vi "Check_Execution_Row.vi"(0 "Execution Row":T1 {"Carrier_2 Q (l/min)" format="%#.2f"; "Row Duration (mins)" format="%#.1f"; "Row No" min=0; "Trace Gas Concentration (%)" min=0.0 format="%#_4f"; "Carrier_1 Q (l/min)" format="%#.4f"; "Start X" format="%#.2f"; "Start Y" format="%#.2f"; "Start Z" format="%#.2f"; "End X" format="%#.2f"; "End Y" format="%#.2f"; "End Z" format="%#.2f"; "Tunnel Speed" format="%#.2f"; "Averaging time (mins)" min=0.0 format="%#.2f"}, 1 "Earlier Filenames":path[](array[path]), 2 "multirunFilepath":path, 3 "Synchronization Start No":i32=1 min=1 max=100, 4 "Row Index":i32, 5 "Max Tunnel Speed":dbl format="%.2f") -> (6 "Edited Row":bool, 7 "Execution Row Out":T1 {"Carrier_2 Q (l/min)" format="%#.2f"; "Row Duration (mins)" format="%#.1f"; "Row No" min=0; "Trace Gas Concentration (%)" min=0.0 format="%#_4f"; "Carrier_1 Q (l/min)" format="%#.4f"; "Start X" format="%#.2f"; "Start Y" format="%#.2f"; "Start Z" format="%#.2f"; "End X" format="%#.2f"; "End Y" format="%#.2f"; "End Z" format="%#.2f"; "Tunnel Speed" format="%#.2f"; "Averaging time (mins)" min=0.0 format="%#.2f"}, 9 "Continue?":bool, 10 "Error Comments":string)   [LabVIEW 2022 SP3]
uses:
  Traverse_cluster.ctl
  Spacing.ctl
  Controls/Multi_run_mode.ctl
  Controls/User_Specific_mode.ctl
  Controls/Home.ctl
  Controls/Tunnel_Coordinates.ctl
  ADAM Client/Sub VIs/ADAM Controls/Channel_names.ctl
  <vilib>/Utility/error.llb/Trim Whitespace One-Sided.vi
  Globals/Extra_Commands_Global.vi
  Globals/Constants_global.vi
  Globals/Trav_pos_global.vi
  Globals/Preference_global.vi
panel:
  out "Traverse line Out":T1 {"Carrier_2 Q (l/min)" format="%#.2f"; "Row Duration (mins)" format="%#.1f"; "Row No" min=0; "Trace Gas Concentration (%)" min=0.0 format="%#_4f"; "Carrier_1 Q (l/min)" format="%#.4f"; "Start X" format="%#.2f"; "Start Y" format="%#.2f"; "Start Z" format="%#.2f"; "End X" format="%#.2f"; "End Y" format="%#.2f"; "End Z" format="%#.2f"; "Tunnel Speed" format="%#.2f"; "Averaging time (mins)" min=0.0 format="%#.2f"}
  out "Fixed Axis":bool[](array[boolean])
  out "Filenames":string[](array[string])
  out "Current Sync Number":i32
  out "Checks":string[](array[string])
  in  "Edit in Excel":bool
  in  "OK":bool
  # "X           Y          Z"
  # "Start"
  # "End"
  # "X           Y          Z"
  # "Start"
  # "End"
  # "X           Y          Z"
  # "Start"
  # "End"
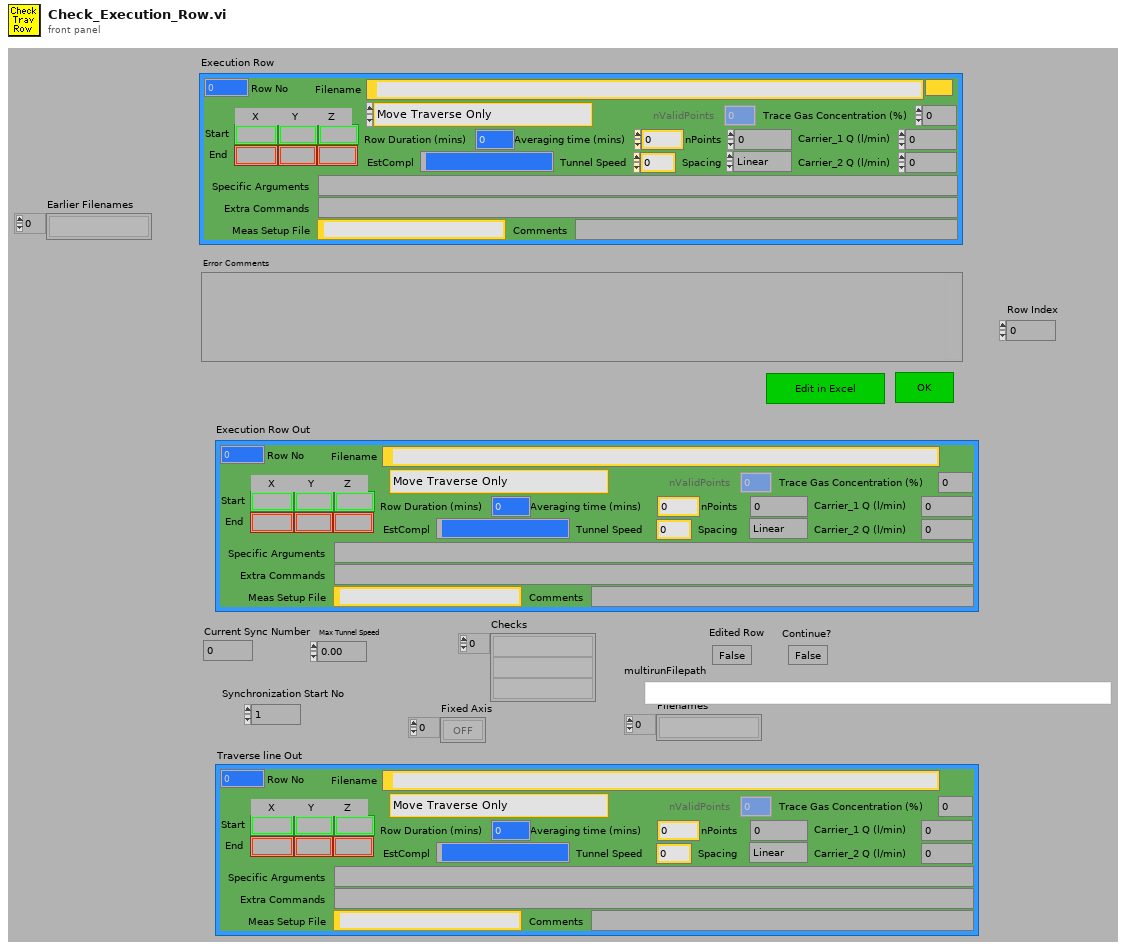
[diagram p1: front panel]
types:
  T1 = typedef "Traverse_cluster.ctl" = cluster{"Start X":sgl, "Start Y":sgl, "Start Z":sgl, "End X":sgl, "End Y":sgl, "End Z":sgl, "nPoints":i32, "Spacing":T2, "Filename":path, "Tunnel Speed":dbl, "Averaging time (mins)":dbl, "Extra Commands":string, "Carrier_1 Q (l/min)":dbl, "Carrier_2 Q (l/min)":dbl, "Trace Gas Concentration (%)":dbl, "Specific Arguments":string, "Comments":string, "Row No":i32, "Row Type Selector":T3, "EstCompl":string, "Row Duration (mins)":dbl, "nValidPoints":i32, "Meas Setup File":string}
  T2 = typedef "Spacing.ctl" = enum16{"Linear", "Log", "Gauss", "Specified", "N/A"}
  T3 = typedef "Multi_run_mode.ctl" = enum16{"Move Traverse Only", "Set Tunnel Speed Only", "Set Source Only", "Set Measurement Conditions", "Single Measurement", "Vertical Profile", "Lateral Profile", "Longitudinal Profile", "Multi-Axis Profile", "Explore Volume", "Auto Calibrate", "Meas Fast FID Bkgnd", "Check Beam Power", "Scanning Valve Measurement", "Run VI Named:", "Set ADAM Ch", "Wait (minutes)", "Send Message", "Synchronize With:", "Fall Back to this Row", "Turn Off Row Repeating", "Traverse 3D Volume", "Blank Row", "Jump to Fall Back Row"}
  T4 = enum16{"All Channel Names", "Valid Channel Names"}
  T5 = typedef "User_Specific_mode.ctl" = enum16{"Check VI only", "Run VI"}
  T6 = typedef "Home.ctl" = enum16{"Don't Home", "Home  +X", "Home  -X", "Home  +Y", "Home  -Y", "Home  +Z", "Home  -Z"}
  T7 = typedef "Tunnel_Coordinates.ctl" = enum16{"Work in Tunnel Coordinates", "Work in Model Coordinates"}
  T8 = enum16{"Zero or one", "One", "Zero or more", "One or more"}
  T9 = typedef "Channel_names.ctl" = enum16{"Active Only", "Active + Off", "All Channels", "Changeable Only", "Always Off", "Always On", "Always Off or On"}
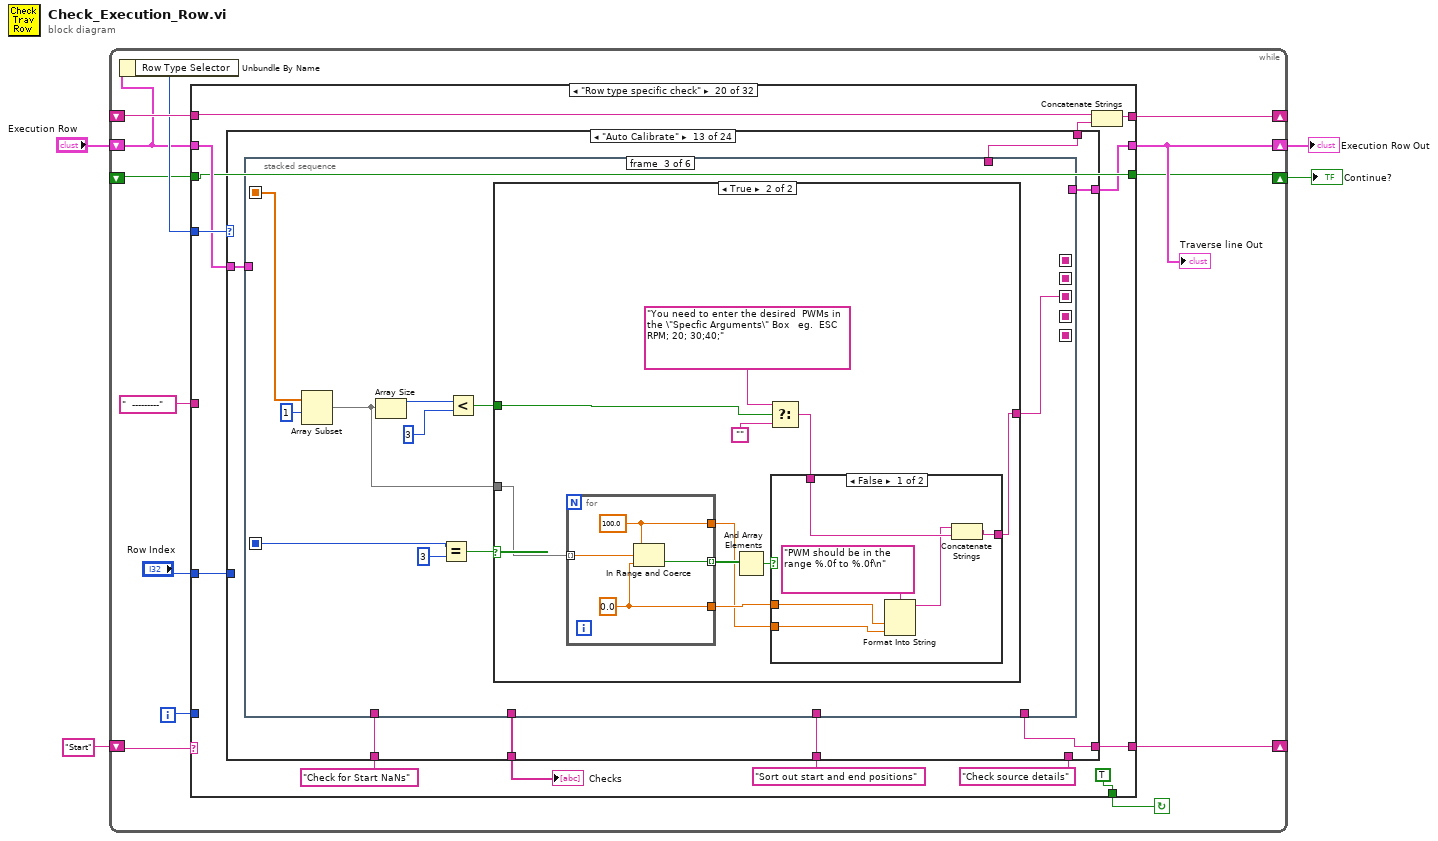
[diagram p0: block diagram]
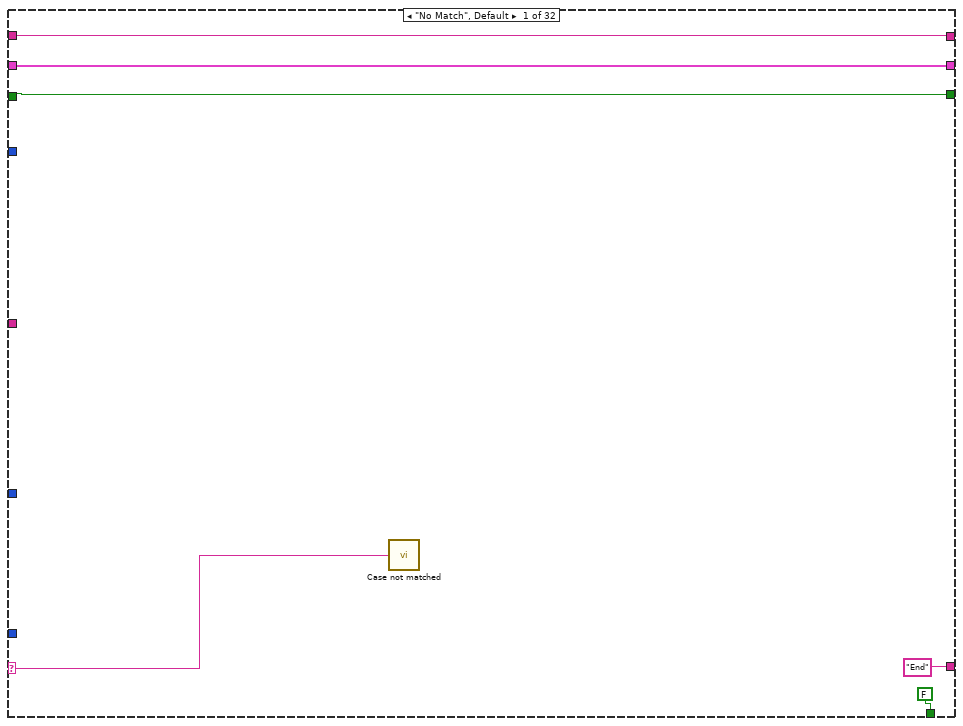
[diagram p2: hidden frame]
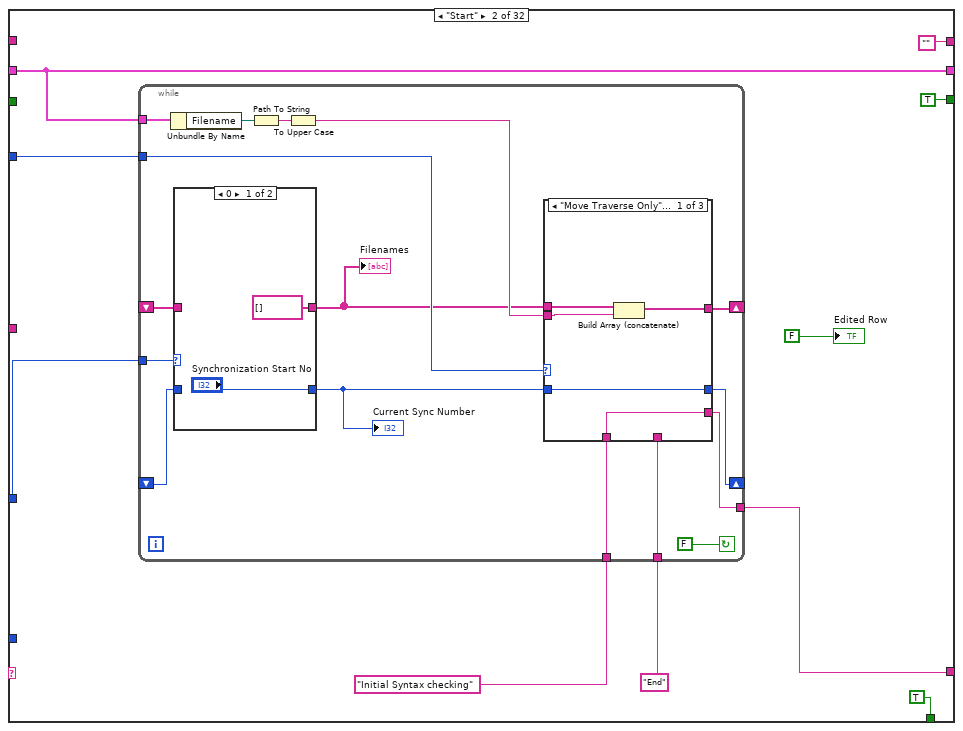
[diagram p3: hidden frame]
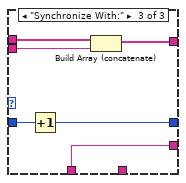
[diagram p6: hidden frame]
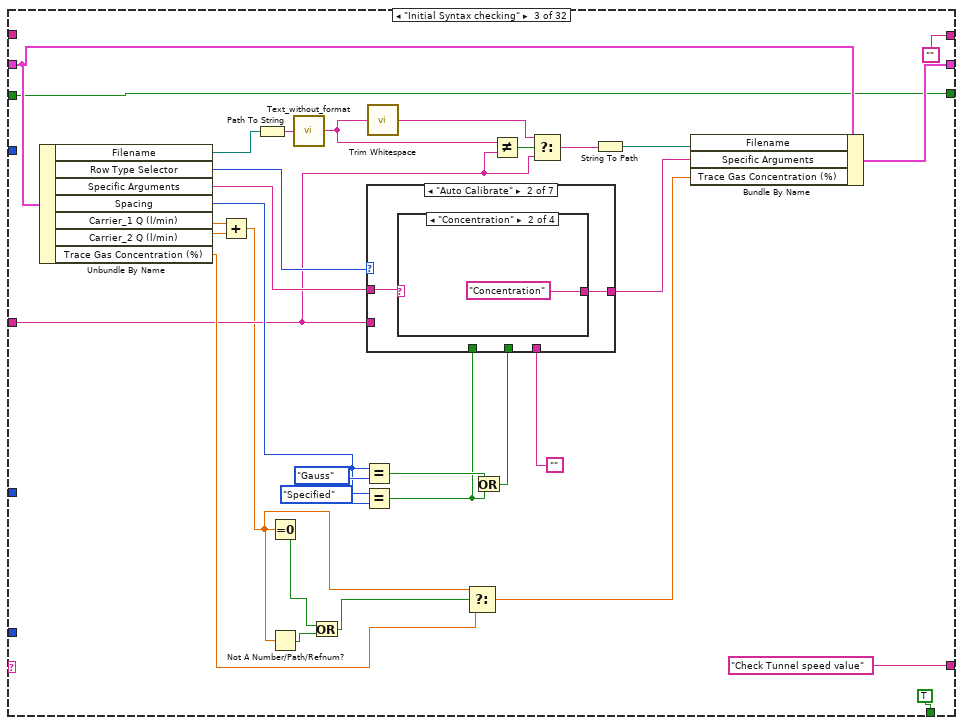
[diagram p7: hidden frame]
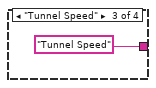
[diagram p10: hidden frame]
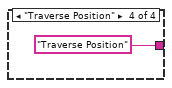
[diagram p11: hidden frame]
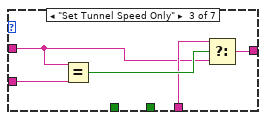
[diagram p12: hidden frame]
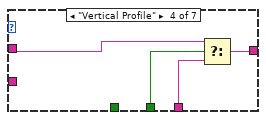
[diagram p13: hidden frame]
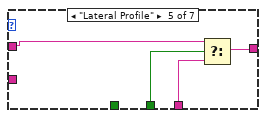
[diagram p14: hidden frame]
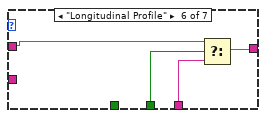
[diagram p15: hidden frame]
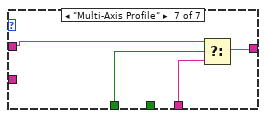
[diagram p16: hidden frame]
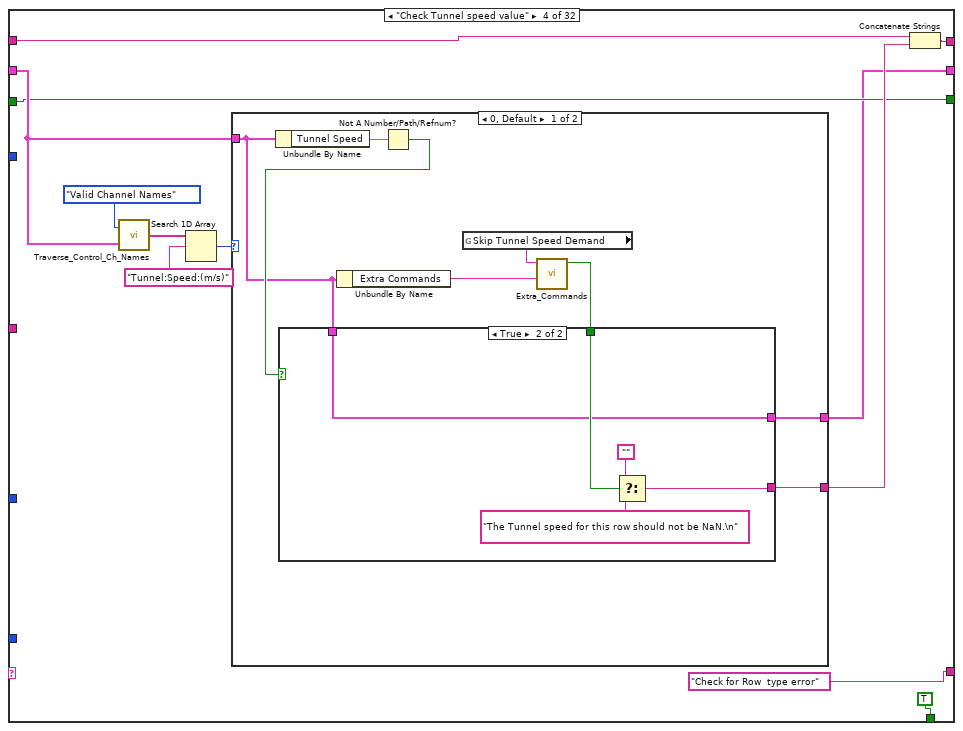
[diagram p17: hidden frame]
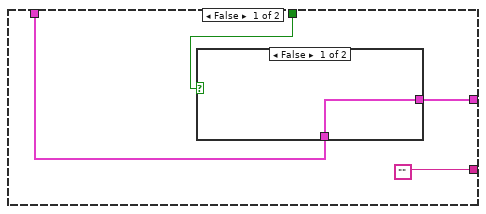
[diagram p18: hidden frame]
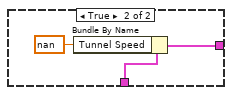
[diagram p19: hidden frame]
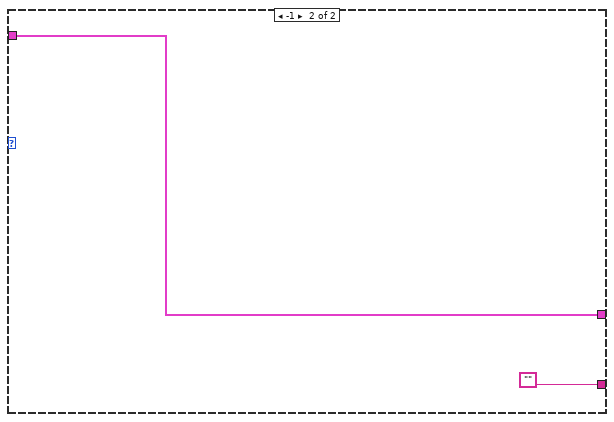
[diagram p20: hidden frame]
diagram:
  n1 = while {
    shift-left: _ -> [w16]
    shift-right: [w17] -> _
    shift-left: "Start" -> [w9]
    shift-right: [w14] -> _
    shift-right: [w8] -> w2
    shift-left: "Execution Row" -> [w5]
    shift-right: [w7] -> w1
    shift-left: _ -> [w6]
    i -> [w10]
    stop <- w15 continue-if-true
    n2 = Unbundle By Name(w5) -> ("Row Type Selector"=w12:T3)
    n3 = case shown="\"Row type specific check\"" w9 {
      tunnel: w5 -> [w23 w27 w94 w132 w166 w198 w223 w272 w302 w332 w363 w389 w422 w499 w526 w565 w620 w652 w660 w699 w1158 w1259 w1291 w1322 w1395 w1403 w1421 w1494 _ w1535 w1542 w1552]
      tunnel: "  ---------" ("f") -> [_ _ w72 _ _ w202 _ _ _ _ _ _ _ _ _ _ _ _ _ _ _ _ _ _ _ _ _ _ _ _ _ _]
      tunnel: "Row Index" -> [_ w31 _ _ _ _ w220 _ _ _ _ _ _ _ _ _ _ _ _ w693 _ _ _ _ _ _ _ _ _ w1536 _ w1551]
      selector: w9 -> [w18 _ _ _ _ _ _ _ _ _ _ _ _ _ _ _ _ _ _ _ _ _ _ _ _ _ _ _ _ _ _ _]
      tunnel: [w22 "" "" w133 w163 w191 w229 w273 w303 w333 w364 w390 w424 w503 w529 w570 w622 w656 w665 w703 w1163 w1269 w1297 w1344 w1394 w1404 w1422 w1500 w1511 w1537 w1547 w1554] -> w17
      tunnel: w12 -> [_ w30 _ _ _ w184 _ _ _ _ _ _ _ _ _ _ _ _ w663 w702 w1159 _ _ _ _ _ w1426 _ _ _ _ _]
      tunnel: w16 -> [w22 _ _ w134 w164 w193 w230 w274 w304 w334 w365 w391 w425 w504 w530 w571 w622 w655 w666 w704 w1163 w1270 w1298 w1345 w1394 w1405 w1427 w1500 w1511 w1537 w1547 w1554]
      tunnel: [FALSE TRUE TRUE TRUE TRUE TRUE TRUE TRUE TRUE TRUE TRUE TRUE TRUE TRUE TRUE TRUE TRUE TRUE TRUE TRUE TRUE TRUE TRUE TRUE TRUE TRUE w1418 TRUE TRUE TRUE TRUE FALSE] -> w15
      tunnel: ["End" w28 "Check Tunnel speed value" ("f") "Check for Row  type error" ("f") "Check Pause syntax" ("f") w196 "Check !Gas Line Name" ("f") "Check !Use_Axis_Correction" ("f") "Check !Use_2D_Offset_for_Axes" ("f") "Check !Offset dx;dy;dz in Tunnel Coord" ("f") "Check !Offset dx;dy;dz in Model Coord" ("f") "Check Traverse Setup Name" ("f") "Check Datum Image Extra command" ("f") "Check Trav_Profile_Plug_In" ("f") "Check IF command" ("f") "Check Measurement Setup?" ("f") w624 "Check Maximum tunnel speed" ("f") "Row type specific check" ("f") w700 "Check for position NaNs" ("f") w1260 "Check source details" ("t") "Check source details" ("f") w1391 "check entered filename etc" ("f") w1424 "What to do next?" ("f") w1509 "Initial Syntax checking" "End" "End"] -> w14
      tunnel: w10 -> [_ _ _ _ _ _ _ _ _ _ _ _ _ _ _ _ _ _ _ _ _ _ _ _ _ _ _ _ _ _ _ _]
      tunnel: [w23 w27 w75 w128 w167 w186 w222 w272 w302 w332 w363 w389 w422 w499 w526 w565 w620 w651 w660 w694 w1157 w1259 w1291 w1321 w1395 w1403 w1420 w1494 w1504 w1538 w1542 w1550] -> w8
      tunnel: [w19 TRUE w73 w131 w173 w187 w224 w271 w301 w331 w362 w388 w420 w497 w525 w562 w626 w653 w658 w696 w1155 w1258 w1290 w1319 w1396 w1401 w1418 w1493 w1503 w1532 w1541 w1548] -> w7
      tunnel: w6 -> [w19 _ w73 w131 w173 w187 w224 w271 w301 w331 w362 w388 w420 w497 w525 w562 w626 w653 w658 w696 w1155 w1258 w1290 w1319 w1396 w1401 _ w1493 _ w1532 w1541 w1548]
      frame "No Match", Default {
        n4 = call "Case not matched.vi"("Case Name not Matched"=w18) -> ()
      }
      frame "Start" {
        n5 = while {
          tunnel: "End" -> [w35]
          tunnel: "Initial Syntax checking" -> [w36]
          tunnel: [w37] -> w28
          tunnel: w27 -> [w44]
          shift-left: _ -> [w43]
          shift-right: [w42] -> _
          tunnel: w30 -> [w48]
          shift-left: _ -> [w47]
          shift-right: [w46] -> _
          tunnel: w31 -> [w49]
          stop <- FALSE continue-if-true
          n6 = Unbundle By Name(w44) -> ("Filename"=w41:path)
          n7 = case shown="0" w49 {
            tunnel: ["Synchronization Start No" w53] -> w45
            tunnel: w47 -> [_ w53]
            tunnel: w43 -> [_ w52]
            tunnel: [string[] [] w52] -> w38
            frame 0 {
            }
            frame 1, Default {
            }
          }
          "Current Sync Number" <- w45
          "Filenames" <- w38
          n8 = Path To String(path=w41) -> (string=w40:string)
          n9 = To Upper Case(1:w40) -> (0:w39:string)
          n10 = case shown="\"Move Traverse Only\", Default" w48 {
            tunnel: w45 -> [w58 w61 w67]
            tunnel: [w58 w61 w66] -> w46
            tunnel: w39 -> [w56 _ w65]
            tunnel: w38 -> [w57 w60 w64]
            tunnel: [w55 w60 w63] -> w42
            tunnel: [w54 w59 w62] -> w37
            tunnel: w36 -> [w54 _ w62]
            tunnel: w35 -> [_ w59 _]
            frame "Move Traverse Only", Default {
              n11 = Build Array (concatenate)(w57, w56) -> (w55:string[])
            }
            frame "Blank Row" {
            }
            frame "Synchronize With:" {
              n12 = Increment(x=w67) -> (x+1=w66:i32)
              n13 = Build Array (concatenate)(w64, w65) -> (w63:string[])
            }
          }
        }
        "Edited Row" <- FALSE ("Editted Row")
      }
      frame "Initial Syntax checking" {
        n14 = Unbundle By Name(w94) -> ("Filename"=w71:path, "Row Type Selector"=w92:T3, "Specific Arguments"=w90:string, "Spacing"=w82:T2, "Carrier_1 Q (l/min)"=w70:dbl, "Carrier_2 Q (l/min)"=w69:dbl, "Trace Gas Concentration (%)"=w88:dbl)
        n15 = Add(x=w70, y=w69) -> (x+y=w68:dbl)
        n16 = Path To String(path=w71) -> (string=w77:string)
        n17 = Equal To 0?(x=w68) -> (x = 0?=w80:bool)
        n18 = Not A Number/Path/Refnum?(number/path/refnum=w68) -> (NaN/Path/Refnum?=w79:bool)
        n19 = call "Text_without_format.vi"("Input string"=w77) -> ("Output string"=w98:string)
        n20 = Or(x=w80, y=w79) -> (x .or. y?=w78:bool)
        n21 = Equal?(x=w82, y=Spacing."Gauss" ("Spacing")) -> (x = y?=w84:bool)
        n22 = Equal?(x=w82, y=Spacing."Specified" ("Spacing")) -> (x = y?=w81:bool)
        n23 = call <vilib>:"Trim Whitespace.vi"("string"=w98) -> ("trimmed string"=w97:string)  [unwired: 1 in]
        n24 = Select(t=w68, s=w78, f=w88) -> (s? t:f=w87:dbl)
        n25 = Or(x=w84, y=w81) -> (x .or. y?=w83:bool)
        n26 = case shown="\"Auto Calibrate\"" w92 {
          tunnel: [w100 w102 w107 w113 w117 w121 w125] -> w91
          tunnel: w90 -> [w100 w101 w108 w115 w119 w123 w127]
          tunnel: "" -> [_ _ w109 w114 w118 w122 w126]
          tunnel: w83 -> [_ _ _ w112 w116 w120 _]
          tunnel: w81 -> [_ _ _ _ _ _ w124]
          tunnel: w72 -> [_ _ w111 _ _ _ _]
          frame "Move Traverse Only", Default {
          }
          frame "Auto Calibrate" {
            n27 = case shown="\"Concentration\"" w101 {
              selector: w101 -> [w103 _ _ _]
              tunnel: [w103 "Concentration" "Tunnel Speed" "Traverse Position"] -> w102
              frame "No Match", Default {
              }
              frame "Concentration" {
              }
              frame "Tunnel Speed" {
              }
              frame "Traverse Position" {
              }
            }
          }
          frame "Set Tunnel Speed Only" {
            n28 = Equal?(x=w108, y=w111) -> (x = y?=w110:bool)
            n29 = Select(t=w109, s=w110, f=w108) -> (s? t:f=w107:string)
          }
          frame "Vertical Profile" {
            n30 = Select(t=w115, s=w112, f=w114) -> (s? t:f=w113:string)
          }
          frame "Lateral Profile" {
            n31 = Select(t=w119, s=w116, f=w118) -> (s? t:f=w117:string)
          }
          frame "Longitudinal Profile" {
            n32 = Select(t=w123, s=w120, f=w122) -> (s? t:f=w121:string)
          }
          frame "Multi-Axis Profile" {
            n33 = Select(t=w127, s=w124, f=w126) -> (s? t:f=w125:string)
          }
        }
        n34 = Not Equal?(x=w98, y=w72) -> (x != y?=w99:bool)
        n35 = Select(t=w97, s=w99, f=w72) -> (s? t:f=w96:string)
        n36 = String To Path(string=w96) -> (path=w76:path)
        n37 = Bundle By Name(cluster=w94, "Filename"=w76, "Specific Arguments"=w91, "Trace Gas Concentration (%)"=w87) -> (w75:T1)
      }
      frame "Check Tunnel speed value" {
        n38 = call "Traverse_Control_Ch_Names.vi"("Traverse line"=w132, "Mode"=T4."Valid Channel Names") -> ("Channel names"=w138:string[])
        n39 = Search 1D Array(1D array=w138, element="Tunnel:Speed:(m/s)" ("Label for value")) -> (index of element=w136:i32)  [unwired: 1 out]
        n40 = case shown="0, Default" w136 {
          tunnel: w132 -> [w141 w161]
          tunnel: [w145 ""] -> w135
          tunnel: [w140 w161] -> w128
          frame 0, Default {
            n41 = Unbundle By Name(w141) -> ("Tunnel Speed"=w147:dbl)
            n42 = Unbundle By Name(w141) -> ("Extra Commands"=w144:string)
            n43 = Not A Number/Path/Refnum?(number/path/refnum=w147) -> (NaN/Path/Refnum?=w146:bool)
            n44 = global read "Extra_Commands_Global.vi" "Skip Tunnel Speed Demand"() -> (w143:string)
            n45 = call "Extra_Commands.vi"("String to Search"=w144, "Command"=w143) -> ("Command Found"=w142:bool)  [unwired: 1 in, 4 out]
            n46 = case shown="True" w146 {
              tunnel: ["" w158] -> w145
              tunnel: w142 -> [w149 w157]
              tunnel: w141 -> [w150 w156]
              tunnel: [w148 w156] -> w140
              frame False {
                n47 = case shown="False" w149 {
                  tunnel: w150 -> [w152 w155]
                  tunnel: [w152 w153] -> w148
                  frame False {
                  }
                  frame True {
                    n48 = Bundle By Name(cluster=w155, "Tunnel Speed"=nan) -> (w153:T1)
                  }
                }
              }
              frame True {
                n49 = Select(t="", s=w157, f="The Tunnel speed for this row should not be NaN.\n") -> (s? t:f=w158:string)
              }
            }
          }
          frame -1 {
          }
        }
        n50 = Concatenate Strings(w134, w135) -> (w133:string)
      }
      frame "Check for Row  type error" {
        n51 = Unbundle By Name(w166) -> ("EstCompl"=w169:string)
        n52 = Match Pattern(string=w169, regular expression="ROW TYPE ERROR " ("format string")) -> (after substring=w168:string, offset past match=w165:i32)  [unwired: 3 out]
        n53 = case shown="0, Default" w165 {
          tunnel: w168 -> [w180 _]
          tunnel: [w178 w182] -> w167
          tunnel: w166 -> [w177 w182]
          tunnel: [w175 w181] -> w163
          tunnel: w164 -> [w174 w181]
          frame 0, Default {
            n54 = Format Into String(format string="The code has guessed the row type from your input string of \"%s\"\nPlease change if this is not the row type that you intended.\n", initial string=w174, w180) -> (resulting string=w175:string)  [unwired: 1 in, 1 out]
            n55 = Bundle By Name(cluster=w177, "EstCompl"="") -> (w178:T1)
          }
          frame -1 {
          }
        }
      }
      frame "Check Pause syntax" {
        n56 = Unbundle By Name(w198) -> ("Extra Commands"=w203:string)
        n57 = Equal?(x=Multi_run_mode."Set ADAM Ch" ("Row Type Selector"), y=w184) -> (x = y?=w183:bool)
        n58 = Not Equal?(x=w203, y=w202) -> (x != y?=w204:bool)
        n59 = Select(t=w203, s=w204, f="") -> (s? t:f=w200:string)
        n60 = call <vilib>:"Trim Whitespace.vi"("string"=w200) -> ("trimmed string"=w195:string)  [unwired: 1 in]
        n61 = case shown="False" w183 {
          tunnel: [w206 TRUE] -> w197
          tunnel: w195 -> [w205 _]
          frame False {
            n62 = Equal?(x=w205, y="") -> (x = y?=w206:bool)
          }
          frame True {
          }
        }
        n63 = call "Pause_for_server_ch_val.vi"("Extra command string"=w195, "Simulate/Run"=User_Specific_mode."Check VI only") -> ("Extra command string Out"=w194:string, "Error Comments"=w192:string)
        n64 = Bundle By Name(cluster=w198, "Extra Commands"=w194) -> (w186:T1)
        n65 = Concatenate Strings(w193, w192) -> (w191:string)
        n66 = Select(t="Check Measurement Setup?", s=w197, f="Check Extra Commands") -> (s? t:f=w196:string)
      }
      frame "Check Extra Commands" {
        n67 = global read "Extra_Commands_Global.vi" "Home"() -> (w209:string)
        n68 = Unbundle By Name(w223) -> ("Extra Commands"=w215:string)
        n69 = for {
          N: 5 -> [_]
          tunnel: w215 -> [w248]
          shift-right: [w244] -> w210
          shift-left: "" -> [w245]
          i -> [w250]
          n70 = case shown="4" w250 {
            tunnel: [w253 w255 w257 w259 w261] -> w247
            tunnel: ["The Extra Command \"%s\" should have a numeric argument of (Centre; Intensity) eg 0 ; 0.85 for Gaussian spacing or (Offset) eg 300 for Log \n" ("Format String") "The Extra Command \"%s\" should have a numeric argument.\n" ("Format String") "The Extra Command \"%s\" should have a numeric argument.\n" ("Format String") "The Extra Command \"%s\" should have a numeric argument.\n" ("Format String") "The Extra Command \"%s\" should have a numeric argument greater than Zero.\n" ("Format String")] -> w242
            frame 0, Default {
              n71 = global read "Extra_Commands_Global.vi" "Point Spacing Parameters"() -> (w253:string)
            }
            frame 1 {
              n72 = global read "Extra_Commands_Global.vi" "Establish Exp Conditions (s)"() -> (w255:string)
            }
            frame 4 {
              n73 = global read "Extra_Commands_Global.vi" "!Traverse Speed Factor"() -> (w257:string)
            }
            frame 2 {
              n74 = global read "Extra_Commands_Global.vi" "Minutes Before Repeating Row"() -> (w259:string)
            }
            frame 3 {
              n75 = global read "Extra_Commands_Global.vi" "Puff Duration Sec"() -> (w261:string)
            }
          }
          n76 = call "Extra_Commands.vi"("String to Search"=w248, "Command"=w247) -> ("String Value"=w249:string, "Command Found"=w251:bool)  [unwired: 1 in, 3 out]
          n77 = case shown="True" w251 {
            tunnel: w249 -> [_ w270]
            tunnel: w247 -> [_ w268]
            tunnel: [w262 w265] -> w246
            tunnel: "" -> [w262 w264]
            tunnel: w242 -> [_ w263]
            frame False {
            }
            frame True {
              n78 = Decimal String To Number(string=w270) -> (offset past number=w269:i32)  [unwired: 3 out]
              n79 = Equal To 0?(x=w269) -> (x = 0?=w267:bool)
              n80 = Format Into String(format string=w263, w268) -> (resulting string=w266:string)  [unwired: 2 in, 1 out]
              n81 = Select(t=w266, s=w267, f=w264) -> (s? t:f=w265:string)
            }
          }
          n82 = Concatenate Strings(w246, w245) -> (w244:string)
        }
        n83 = call "Extra_Commands.vi"("String to Search"=w215, "Command"=w209) -> ("String Value"=w213:string, "Command Found"=w214:bool)  [unwired: 1 in, 3 out]
        n84 = case shown="True" w214 {
          tunnel: w213 -> [_ w241]
          tunnel: [TRUE w238] -> w212
          frame False {
          }
          frame True {
            n85 = call "Home_String_to_Enumerated_Type.vi"("String"=w241) -> ("Home"=w240:T6)
            n86 = Not Equal?(x=w240, y=Home."Don't Home" ("Home")) -> (x != y?=w238:bool)
          }
        }
        n87 = call "Trav_Prog_Extra_Commands.vi"() -> ("Extra Commands Array"=w225:string[])  [unwired: 2 out]
        n88 = call "Valid_Extra_Command.vi"("Extra Commands string"=w215, "Valid Commands Array"=w225) -> ("Output String"=w228:string, "Extra Commands string Out"=w221:string)  [unwired: 3 out]
        n89 = Bundle By Name(cluster=w223, "Extra Commands"=w221) -> (w222:T1)
        n90 = call "Skip_If Sd_Error_Below.vi"("String to Search"=w221, "Simulate/Run"=User_Specific_mode."Check VI only", "Measurement setup Applied?"=FALSE, "Row Number"=w220) -> ("Error String"=w217:string)  [unwired: 1 in, 4 out]
        n91 = case shown="False" w212 {
          tunnel: [w234 w236] -> w211
          tunnel: w210 -> [w233 w236]
          tunnel: w209 -> [w235 _]
          frame False {
            n92 = Format Into String(format string="The Extra Command \"%s\" argument should be either\nHome  +X\nHome  -X\nHome  +Y\nHome  -Y\nHome  +Z\nHome  -Z\n" ("Format String"), initial string=w233, w235) -> (resulting string=w234:string)  [unwired: 1 in, 1 out]
          }
          frame True {
          }
        }
        n93 = Concatenate Strings(w230, w228, w211, w217) -> (w229:string)
      }
      frame "Check !Gas Line Name" {
        n94 = Unbundle By Name(w272) -> ("Extra Commands"=w280:string)
        n95 = global read "Extra_Commands_Global.vi" "Gas Line Name"() -> (w275:string)
        n96 = call "Extra_Commands.vi"("String to Search"=w280, "Command"=w275) -> ("String Value"=w276:string, "Command Found"=w277:bool)  [unwired: 1 in, 3 out]
        n97 = case shown="True" w277 {
          tunnel: w276 -> [_ w285]
          tunnel: w275 -> [_ w288]
          tunnel: w274 -> [w281 w287]
          tunnel: [w281 w286] -> w273
          frame False {
          }
          frame True {
            n98 = call "Gas Line Names.vi"() -> ("Gas line Names"=w282:string[])  [unwired: 5 in]
            n99 = Search 1D Array(1D array=w282, element=w285) -> (index of element=w284:i32)  [unwired: 1 in]
            n100 = Greater Or Equal To 0?(x=w284) -> (x >= 0?=w283:bool)
            n101 = case shown="False" w283 {
              tunnel: [w294 w300] -> w286
              tunnel: w287 -> [w293 w300]
              tunnel: w288 -> [w295 _]
              tunnel: w282 -> [w290 _]
              frame False {
                n102 = for {
                  shift-right: [w297] -> w289
                  shift-left: "" -> [w299]
                  tunnel: w290 -> [w296] mode=indexing
                  n103 = Concatenate Strings(w299, w296, "\r\n") -> (w297:string)
                }
                n104 = Format Into String(format string="The Extra Command \"%s\" argument must be one of the following:\n%s" ("Format String"), initial string=w293, w295, w289) -> (resulting string=w294:string)  [unwired: 1 in, 1 out]
              }
              frame True {
              }
            }
          }
        }
      }
      frame "Check !Use_Axis_Correction" {
        n105 = Unbundle By Name(w302) -> ("Extra Commands"=w310:string)
        n106 = global read "Extra_Commands_Global.vi" "!Use_Axis_Correction"() -> (w305:string)
        n107 = call "Extra_Commands.vi"("String to Search"=w310, "Command"=w305) -> ("String Value"=w306:string, "Command Found"=w307:bool)  [unwired: 1 in, 3 out]
        n108 = case shown="True" w307 {
          tunnel: w306 -> [_ w321]
          tunnel: w305 -> [_ w315]
          tunnel: w304 -> [w311 w314]
          tunnel: [w311 w313] -> w303
          frame False {
          }
          frame True {
            n109 = call "Get_array_values_fr_String.vi"("String Value"=w321) -> ("String array"=w320:string[])  [unwired: 1 out]
            n110 = Build Array("X", "Y", "Z") -> (w316:string[])
            n111 = for {
              tunnel: w320 -> [w330] mode=indexing
              tunnel: w316 -> [w329]
              tunnel: [w327] -> w312
              stop <- w327 continue-if-true
              n112 = Search 1D Array(1D array=w329, element=w330) -> (index of element=w328:i32)  [unwired: 1 in]
              n113 = Greater Or Equal To 0?(x=w328) -> (x >= 0?=w327:bool)
            }
            n114 = case shown="False" w312 {
              tunnel: [w324 w326] -> w313
              tunnel: w314 -> [w323 w326]
              tunnel: w315 -> [w325 _]
              frame False {
                n115 = Format Into String(format string="The Extra Command \"%s\" argument is invalid Example\n !Use_Axis_Correction = Y" ("Format String"), initial string=w323, w325) -> (resulting string=w324:string)  [unwired: 1 in, 1 out]
              }
              frame True {
              }
            }
          }
        }
      }
      frame "Check !Use_2D_Offset_for_Axes" {
        n116 = Unbundle By Name(w332) -> ("Extra Commands"=w340:string)
        n117 = global read "Extra_Commands_Global.vi" "!Use_2D_Offset_for_Axes"() -> (w335:string)
        n118 = call "Extra_Commands.vi"("String to Search"=w340, "Command"=w335) -> ("String Value"=w336:string, "Command Found"=w337:bool)  [unwired: 1 in, 3 out]
        n119 = case shown="True" w337 {
          tunnel: w336 -> [_ w351]
          tunnel: w335 -> [_ w345]
          tunnel: w334 -> [w341 w344]
          tunnel: [w341 w343] -> w333
          frame False {
          }
          frame True {
            n120 = call "Get_array_values_fr_String.vi"("String Value"=w351) -> ("String array"=w350:string[])  [unwired: 1 out]
            n121 = Build Array("X", "Y", "Z") -> (w346:string[])
            n122 = for {
              tunnel: w350 -> [w360] mode=indexing
              tunnel: w346 -> [w359]
              tunnel: [w357] -> w342
              stop <- w357 continue-if-true
              n123 = Search 1D Array(1D array=w359, element=w360) -> (index of element=w358:i32)  [unwired: 1 in]
              n124 = Greater Or Equal To 0?(x=w358) -> (x >= 0?=w357:bool)
            }
            n125 = case shown="False" w342 {
              tunnel: [w354 w356] -> w343
              tunnel: w344 -> [w353 w356]
              tunnel: w345 -> [w355 _]
              frame False {
                n126 = Format Into String(format string="The Extra Command \"%s\" argument is invalid Example\n!Use_2D_Offset_for_Axes = Y" ("Format String"), initial string=w353, w355) -> (resulting string=w354:string)  [unwired: 1 in, 1 out]
              }
              frame True {
              }
            }
          }
        }
      }
      frame "Check !Offset dx;dy;dz in Tunnel Coord" {
        n127 = Unbundle By Name(w363) -> ("Extra Commands"=w370:string)
        n128 = global read "Extra_Commands_Global.vi" "!Offset dx;dy;dz in Tunnel Coord"() -> (w366:string)
        n129 = call "Extra_Commands.vi"("String to Search"=w370, "Command"=w366) -> ("String Value"=w367:string, "Command Found"=w368:bool)  [unwired: 1 in, 3 out]
        n130 = case shown="True" w368 {
          tunnel: w367 -> [_ w379]
          tunnel: w366 -> [_ w378]
          tunnel: w365 -> [w371 w377]
          tunnel: [w371 w376] -> w364
          frame False {
          }
          frame True {
            n131 = call "Get_array_values_fr_String.vi"("String Value"=w379) -> ("String array"=w375:string[])  [unwired: 1 out]
            n132 = for {
              N: 3 -> [_]
              tunnel: w375 -> [w386] mode=indexing
              tunnel: [w385] -> w373 mode=indexing
              n133 = Fract/Exp String To Number(string=w386) -> (offset past number=w387:i32)  [unwired: 3 in, 1 out]
              n134 = Greater Than 0?(x=w387) -> (x > 0?=w385:bool)
            }
            n135 = And Array Elements(Boolean array=w373) -> (logical AND=w372:bool)
            n136 = case shown="True" w372 {
              tunnel: [w382 w384] -> w376
              tunnel: w377 -> [w381 w384]
              tunnel: w378 -> [w383 _]
              frame False {
                n137 = Format Into String(format string="The Extra Command \"%s\" argument is invalid Example\n!Offset Position by dx;dy;dz = 0;1;0" ("Format String"), initial string=w381, w383) -> (resulting string=w382:string)  [unwired: 1 in, 1 out]
              }
              frame True {
              }
            }
          }
        }
      }
      frame "Check !Offset dx;dy;dz in Model Coord" {
        n138 = Unbundle By Name(w389) -> ("Extra Commands"=w397:string)
        n139 = global read "Extra_Commands_Global.vi" "!Offset dx;dy;dz in Model Coord"() -> (w392:string)
        n140 = call "Extra_Commands.vi"("String to Search"=w397, "Command"=w392) -> ("String Value"=w393:string, "Command Found"=w394:bool)  [unwired: 1 in, 3 out]
        n141 = case shown="True" w394 {
          tunnel: w393 -> [_ w406]
          tunnel: w392 -> [_ w405]
          tunnel: w391 -> [w398 w404]
          tunnel: [w398 w403] -> w390
          frame False {
          }
          frame True {
            n142 = call "Get_array_values_fr_String.vi"("String Value"=w406) -> ("String array"=w402:string[])  [unwired: 1 out]
            n143 = for {
              N: 3 -> [_]
              tunnel: w402 -> [w413] mode=indexing
              tunnel: [w412] -> w400 mode=indexing
              n144 = Fract/Exp String To Number(string=w413) -> (offset past number=w414:i32)  [unwired: 3 in, 1 out]
              n145 = Greater Than 0?(x=w414) -> (x > 0?=w412:bool)
            }
            n146 = And Array Elements(Boolean array=w400) -> (logical AND=w399:bool)
            n147 = case shown="True" w399 {
              tunnel: [w409 w411] -> w403
              tunnel: w404 -> [w408 w411]
              tunnel: w405 -> [w410 _]
              frame False {
                n148 = Format Into String(format string="The Extra Command \"%s\" argument is invalid Example\n!Offset Position by dx;dy;dz = 0;1;0" ("Format String"), initial string=w408, w410) -> (resulting string=w409:string)  [unwired: 1 in, 1 out]
              }
              frame True {
              }
            }
          }
        }
      }
      frame "Check Traverse Setup Name" {
        n149 = Unbundle By Name(w422) -> ("Extra Commands"=w415:string)
        n150 = global read "Extra_Commands_Global.vi" "!Traverse Setup"() -> (w417:string)
        n151 = call "Extra_Commands.vi"("String to Search"=w415, "Command"=w417) -> ("Command Found"=w416:bool)  [unwired: 1 in, 4 out]
        n152 = case shown="True" w416 {
          tunnel: [w426 w431] -> w421
          tunnel: "" -> [w426 w430]
          tunnel: w415 -> [_ w429]
          frame False {
          }
          frame True {
            n153 = call "Which_Trav_Setup.vi"("Extra Command String"=w429) -> ("Traverse Setups"=w428:string[], "XYZ Offset of 2nd Traverse"=w427:sgl[])  [unwired: 1 out]
            n154 = stacked-sequence {
              seq-local: [w439 _] -> [_ w467]
              tunnel: [_ w466] -> w431
              tunnel: w430 -> [w440 _]
              tunnel: w428 -> [w436 w472]
              tunnel: w427 -> [_ w468]
              frame #0 {
                n155 = global read "Constants_global.vi" "Traverse folder"() -> (w434:path)
                n156 = Empty Array?(array=w436) -> (empty?=w438:bool)
                n157 = Select(t=string[] [""], s=w438, f=w436) -> (s? t:f=w435:string[])
                n158 = call "Get Traverse Names.vi"("Traverse name"="", "Traverse\nSetup\nFolder"=w434) -> ("Traverse Names"=w433:string[])  [unwired: 1 out]
                n159 = for {
                  tunnel: w435 -> [w458] mode=indexing
                  tunnel: w433 -> [w460]
                  shift-right: [w456] -> w442
                  shift-left: w440 -> [w457]
                  n160 = Search 1D Array(1D array=w460, element=w458) -> (index of element=w459:i32)  [unwired: 1 out]
                  n161 = case shown="-1" w459 {
                    tunnel: w458 -> [_ w464]
                    tunnel: [w461 w463] -> w456
                    tunnel: w457 -> [w461 w462]
                    frame Default {
                    }
                    frame -1 {
                      n162 = Format Into String(format string="%s is not a valid Travese setup.\n", initial string=w462, w464) -> (resulting string=w463:string)  [unwired: 1 in, 1 out]
                    }
                  }
                }
                n163 = Empty String/Path?(string/path=w442) -> (empty?=w441:bool)
                n164 = case shown="False" w441 {
                  tunnel: w433 -> [w449 _]
                  tunnel: [w448 w455] -> w439
                  tunnel: w442 -> [w446 w455]
                  frame False {
                    w443 = "\r\n"
                    n165 = Concatenate Strings(w446, " Valid option are:" ("format string"), w443) -> (w445:string)
                    n166 = for {
                      shift-right: [w452] -> w448
                      shift-left: w445 -> [w453]
                      tunnel: w449 -> [w454] mode=indexing
                      tunnel: "!Traverse Setup =  " ("Substring") -> [w451]
                      tunnel: w443 -> [w450]
                      n167 = Concatenate Strings(w453, w451, w454, w450) -> (w452:string)
                    }
                  }
                  frame True {
                  }
                }
              }
              frame #1 {
                n168 = Array Size(array=w472) -> (size(s)=w471:i32)
                n169 = Greater?(x=w471, y=1) -> (0:w469:bool)
                n170 = case shown="True" w469 {
                  tunnel: w468 -> [_ w477]
                  tunnel: w467 -> [w473 w475]
                  tunnel: [w473 w474] -> w466
                  frame False {
                  }
                  frame True {
                    n171 = Array Size(array=w477) -> (size(s)=w478:i32)
                    n172 = case shown="3" w478 {
                      tunnel: w477 -> [_ _ _ w488]
                      tunnel: [FALSE TRUE TRUE w486] -> w476
                      frame 0 {
                      }
                      frame 1, Default {
                      }
                      frame 2 {
                      }
                      frame 3 {
                        n173 = for {
                          tunnel: w488 -> [w490] mode=indexing
                          tunnel: [w489] -> w487 mode=indexing
                          n174 = Not A Number/Path/Refnum?(number/path/refnum=w490) -> (NaN/Path/Refnum?=w489:bool)
                        }
                        n175 = Or Array Elements(Boolean array=w487) -> (logical OR=w486:bool)
                      }
                    }
                    n176 = case shown="True" w476 {
                      tunnel: w475 -> [w479 w482]
                      tunnel: [w479 w480] -> w474
                      frame False {
                      }
                      frame True {
                        n177 = Concatenate Strings(w482, "Invalid offset for the 2nd traverse.\nExample\n!Traverse Setup =  1st Trav; 2nd Trav; Xoffset; Yoffset; Zoffset;  " ("string")) -> (w480:string)
                      }
                    }
                  }
                }
              }
            }
          }
        }
        n178 = Concatenate Strings(w425, w421) -> (w424:string)
      }
      frame "Check Datum Image Extra command" {
        n179 = Unbundle By Name(w499) -> ("Extra Commands"=w496:string)
        n180 = global read "Extra_Commands_Global.vi" "Datum Image"() -> (w501:string)
        n181 = call "Extra_Commands.vi"("String to Search"=w496, "Command"=w501) -> ("String Value"=w493:string, "Command Found"=w500:bool)  [unwired: 1 in, 3 out]
        n182 = call "Get_array_values_fr_String.vi"("String Value"=w493) -> ("String array"=w492:string[])  [unwired: 1 out]
        n183 = Index Array(array=w492) -> (element=w491:string)  [unwired: 1 in]
        n184 = case shown="True" w500 {
          tunnel: w491 -> [_ w511]
          tunnel: [w505 w508] -> w498
          tunnel: "" -> [w505 w507]
          frame False {
          }
          frame True {
            n185 = Build Path(base path=path "hello", name or relative path=w511) -> (appended path=w510:path)
            n186 = call "Current_Filepath.vi"("Short_Name"="Cal" ("Data Type"), "Filename in"=w510, "Data Type"="Calibrations") -> ("Filename Out"=w506:path)  [unwired: 1 in, 1 out]
            n187 = call "Does_file_exist_(simple).vi"("Pathname"=w506) -> ("exists?"=w509:bool)
            n188 = case shown="False" w509 {
              tunnel: [w515 w518] -> w508
              tunnel: w507 -> [_ w518]
              tunnel: w506 -> [w517 _]
              frame False {
                n189 = Format Into String(format string="Cannot find Datum Image File\n%s", w517) -> (resulting string=w515:string)  [unwired: 2 in, 1 out]
              }
              frame True {
              }
            }
          }
        }
        n190 = Concatenate Strings(w504, w498) -> (w503:string)
      }
      frame "Check Trav_Profile_Plug_In" {
        n191 = global read "Extra_Commands_Global.vi" "Trav_Profile_Plug_In"() -> (w527:string)
        n192 = Unbundle By Name(w526) -> ("Extra Commands"=w524:string)
        n193 = call "Extra_Commands.vi"("String to Search"=w524, "Command"=w527) -> ("String Value"=w521:string, "Command Found"=w522:bool)  [unwired: 1 in, 3 out]
        n194 = case shown="True" w522 {
          tunnel: w521 -> [_ w541]
          tunnel: [w531 w538] -> w519
          tunnel: "" -> [w531 w537]
          frame False {
          }
          frame True {
            n195 = call "Get_array_values_fr_String.vi"("String Value"=w541) -> ("String array"=w534:string[])  [unwired: 1 out]
            n196 = Index Array(array=w534) -> (element=w533:string)  [unwired: 1 in]
            n197 = call "Plug_in_Directories.vi"() -> ("Trav_Profile_Plug_Ins"=w536:path)  [unwired: 2 in, 4 out]
            n198 = List Folder(path=w536) -> (filenames=w535:string[])  [unwired: 1 in, 5 out]
            n199 = Search 1D Array(1D array=w535, element=w533) -> (index of element=w532:i32)  [unwired: 1 out]
            n200 = case shown="Default" w532 {
              tunnel: w533 -> [_ w545]
              tunnel: [w542 w544] -> w540
              tunnel: w537 -> [w542 w543]
              frame Default {
              }
              frame -1 {
                n201 = Format Into String(format string="%s is not a valid Trav_Profile_Plug_In name.\n", initial string=w543, w545) -> (resulting string=w544:string)  [unwired: 1 in, 1 out]
              }
            }
            n202 = Empty String/Path?(string/path=w540) -> (empty?=w539:bool)
            n203 = case shown="False" w539 {
              tunnel: w535 -> [w553 _]
              tunnel: [w552 w559] -> w538
              tunnel: w540 -> [w550 w559]
              frame False {
                w547 = "\r\n"
                n204 = Concatenate Strings(w550, " Valid option are:" ("format string"), w547) -> (w549:string)
                n205 = for {
                  shift-right: [w556] -> w552
                  shift-left: w549 -> [w557]
                  tunnel: w553 -> [w558] mode=indexing
                  tunnel: "!Trav_Profile_Plug_In =  " ("Substring") -> [w555]
                  tunnel: w547 -> [w554]
                  n206 = Concatenate Strings(w557, w555, w558, w554) -> (w556:string)
                }
              }
              frame True {
              }
            }
          }
        }
        n207 = Concatenate Strings(w530, w519) -> (w529:string)
      }
      frame "Check IF command" {
        n208 = Unbundle By Name(w565) -> ("Extra Commands"=w561:string)
        n209 = global read "Extra_Commands_Global.vi" "If Command"() -> (w568:string)
        n210 = call "Extra_Commands.vi"("String to Search"=w561, "Command"=w568) -> ("String Value"=w566:string, "Command Found"=w567:bool)  [unwired: 1 in, 3 out]
        n211 = case shown="True" w567 {
          tunnel: w566 -> [_ w577]
          tunnel: [w572 w576] -> w563
          tunnel: "" -> [w572 w574]
          frame False {
          }
          frame True {
            n212 = call "Get_array_values_fr_String.vi"("String Value"=w577) -> ("Numeric Array"=w573:dbl[], "String array"=w575:string[])
            n213 = Index Array(array=w575, index=0 ("Index")) -> (element=w578:string)
            n214 = case shown="\"ADAM Channel Between\"" w578 {
              tunnel: w577 -> [w583 _ _ _]
              tunnel: [w582 w607 w608 "The !If  command has not been recognised.\nExtra command Example:\n!IF = Time Between;10:45;and;14:00;Execute Row (or) Skip Row\n\n!IF = ADAM Channel Between;Channel Name; 0.5;1.0\n\n!IF = Global Value Between; 0.5;1.0" ("Error Comments")] -> w576
              tunnel: w575 -> [_ w600 w616 _]
              tunnel: w574 -> [_ w593 w609 _]
              tunnel: w573 -> [_ _ _ _]
              frame "Time Between" {
                n215 = Get Date/Time In Seconds() -> (seconds since 1Jan1904=w580:timestamp)
                n216 = To Double Precision Float(number=w580) -> (double precision float=w581:dbl)
                n217 = call "If_Time_arguments.vi"("seconds since 1Jan1904"=w581, "String Value"=w583) -> ("Error Comments"=w582:string)  [unwired: 2 out]
              }
              frame "ADAM Channel Between" {
                n218 = Index Array(array=w600, index=1 ("Index")) -> (element=w584:string)
                n219 = Index Array(array=w600, index=2 ("Index")) -> (element=w599:string)
                n220 = Index Array(array=w600, index=3 ("Index")) -> (element=w598:string)
                n221 = Decimal Digit?(1:w599) -> (0:w596:bool)
                n222 = Decimal Digit?(1:w598) -> (0:w597:bool)
                n223 = call "Get_Current_Scan_client.vi"("singleChannel"=w584) -> ("Numerical Values"=w605:dbl[])  [unwired: 1 in, 3 out]
                n224 = And(x=w596, y=w597) -> (x .and. y?=w595:bool)
                n225 = Index Array(array=w605, index=0 ("Index")) -> (element=w606:dbl)
                n226 = Select(t=w593, s=w595, f="you must give two limits\n") -> (s? t:f=w589:string)
                n227 = Not A Number/Path/Refnum?(number/path/refnum=w606) -> (NaN/Path/Refnum?=w592:bool)
                n228 = Select(t="Invalid ADAM Channel Name\n", s=w592, f=w593) -> (s? t:f=w590:string)
                n229 = Concatenate Strings(w590, w589) -> (w587:string)
                n230 = Concatenate Strings(w587, "Extra command Example:\n!IF = ADAM Channel Between;Channel Name; 0.5;1.0") -> (w586:string)
                n231 = Empty String/Path?(string/path=w587) -> (empty?=w588:bool)
                n232 = Select(t=w593, s=w588, f=w586) -> (s? t:f=w607:string)
              }
              frame "Global Value Between" {
                n233 = Index Array(array=w616, index=1 ("Index")) -> (element=w615:string)
                n234 = Index Array(array=w616, index=2 ("Index")) -> (element=w614:string)
                n235 = Decimal Digit?(1:w615) -> (0:w612:bool)
                n236 = Decimal Digit?(1:w614) -> (0:w613:bool)
                n237 = And(x=w612, y=w613) -> (x .and. y?=w611:bool)
                n238 = Select(t=w609, s=w611, f="The Extra command IF statement must have two numerical values for the limits\n\nExtra command Example:\n!IF = Global Value Between; 0.5;1.0") -> (s? t:f=w608:string)
              }
              frame "No Match", Default {
              }
            }
          }
        }
        n239 = Concatenate Strings(w571, w563) -> (w570:string)
      }
      frame "Check Measurement Setup?" {
        n240 = Unbundle By Name(w620) -> ("Row Type Selector"=w625:T3, "Specific Arguments"=w623:string)
        n241 = case shown="\"Run VI Named:\"" w625 {
          tunnel: ["Check Measurement Setup" ("t") "Check Measurement Setup" ("t") "Check Measurement Setup" ("t") "Check Measurement Setup" ("t") "Check Measurement Setup" ("t") "Check Measurement Setup" ("t") "Check Measurement Setup" ("t") "Check Measurement Setup" ("t") "Check Measurement Setup" ("t") "Check Measurement Setup" ("t") w638 w647] -> w624
          tunnel: w623 -> [_ _ _ _ _ _ _ _ _ _ w645 _]
          tunnel: "Check Maximum tunnel speed" ("f") -> [_ _ _ _ _ _ _ _ _ _ w639 w647]
          tunnel: w620 -> [_ _ _ _ _ _ _ _ _ _ w642 _]
          frame "Lateral Profile" {
          }
          frame "Traverse 3D Volume" {
          }
          frame "Longitudinal Profile" {
          }
          frame "Explore Volume" {
          }
          frame "Multi-Axis Profile" {
          }
          frame "Vertical Profile" {
          }
          frame "Single Measurement" {
          }
          frame "Scanning Valve Measurement" {
          }
          frame "Auto Calibrate" {
          }
          frame "Meas Fast FID Bkgnd" {
          }
          frame "Run VI Named:" {
            n242 = Match Pattern(string=w645, regular expression=";") -> (before substring=w644:string)  [unwired: 4 out]
            n243 = call <vilib>:"Trim Whitespace.vi"("string"=w644) -> ("trimmed string"=w643:string)  [unwired: 1 in]
            n244 = call "Run_VI_Named_specific.vi"("Run VI Named String"=w643, "Multi Run Row"=w642) -> ("Check Meas Setup?"=w641:bool)  [unwired: 1 in, 8 out]
            n245 = Select(t="Check Measurement Setup", s=w641, f=w639) -> (s? t:f=w638:string)
          }
          frame "Set Tunnel Speed Only", Default {
          }
        }
      }
      frame "Check Measurement Setup" {
        n246 = Unbundle By Name(w652) -> ("Meas Setup File"=w650:string)
        n247 = call "Check_Measurement_Setups.vi"("Measurement Setup String"=w650) -> ("Measurement Setup String Out"=w649:string, "Error Comments"=w648:string)
        n248 = Bundle By Name(cluster=w652, "Meas Setup File"=w649) -> (w651:T1)
        n249 = Concatenate Strings(w655, w648) -> (w656:string)
      }
      frame "Check Maximum tunnel speed" {
        n250 = case shown="\"Auto Calibrate\"" w663 {
          tunnel: w660 -> [w685 _]
          tunnel: [w676 FALSE] -> w662
          tunnel: [w675 0.0] -> w661
          frame "Auto Calibrate" {
            n251 = Unbundle By Name(w685) -> ("Specific Arguments"=w684:string)
            n252 = call "Get_array_values_fr_String.vi"("String Value"=w684) -> ("Numeric Array"=w678:dbl[], "String array"=w683:string[])
            n253 = Index Array(array=w683, index=0 ("Index")) -> (element=w681:string)
            n254 = Equal?(x=w681, y="Tunnel Speed" ("Output Array")) -> (x = y?=w676:bool)
            n255 = Array Subset(array=w678, index=1 ("Array Index")) -> (w677:dbl[])  [unwired: 1 in]
            n256 = Array Max & Min(array=w677) -> (max value=w675:dbl)  [unwired: 3 out]
          }
          frame "Set Tunnel Speed Only", Default {
          }
        }
        n257 = case shown="False" w662 {
          tunnel: [w673 w674] -> w670
          tunnel: w660 -> [w672 _]
          tunnel: w661 -> [_ w674]
          frame False {
            n258 = Unbundle By Name(w672) -> ("Tunnel Speed"=w673:dbl)
          }
          frame True {
          }
        }
        n259 = Greater?(x=w670, y="Max Tunnel Speed") -> (0:w668:bool)
        n260 = Not A Number/Path/Refnum?(number/path/refnum=w670) -> (NaN/Path/Refnum?=w669:bool)
        n261 = Compound Arithmetic op=AND(invert w669, w668) -> (w667:bool)
        n262 = case shown="True" w667 {
          tunnel: w666 -> [w688 w690]
          tunnel: [w688 w689] -> w665
          tunnel: "Max Tunnel Speed" -> [_ w692]
          frame False {
          }
          frame True {
            n263 = Format Into String(format string="The maximum allowable tunnel speed is %.2f m/s.\n" ("Format String"), initial string=w690, w692) -> (resulting string=w689:string)  [unwired: 1 in, 1 out]
          }
        }
      }
      frame "Row type specific check" {
        n264 = case shown="\"Auto Calibrate\"" w702 {
          tunnel: w699 -> [w714 w725 w738 w742 w746 w751 w756 w763 w770 w798 w809 w824 w830 w969 w974 w978 w1019 w1085 w1113 w1118 w1122 w1134 w1138 w1144]
          tunnel: [string[] [] string[] [] string[] [] string[] [] string[] [] w752 w759 w766 w773 w802 w814 w825 w834 w971 string[] [] w995 string[] [] w1080 string[] [] string[] [] string[] [] string[] [] string[] [] string[] []] -> w701
          tunnel: [w708 w724 "" "" "" "" "" "" "" w781 w811 "" w828 w965 "" w990 w1002 w1096 w1115 "" w1124 "" "" w1146] -> w705
          tunnel: [w716 w731 w739 w743 w747 w750 w757 w764 w771 w797 w810 w823 w832 w959 w975 w989 w1022 w1081 "check entered filename etc" "check entered filename etc" "check entered filename etc" "check entered filename etc" "check entered filename etc" "check entered filename etc"] -> w700
          tunnel: "Check source details" -> [_ w731 w739 w743 _ _ _ _ _ _ _ w823 _ w959 w975 w989 w1021 w1082 _ _ _ _ _ _]
          tunnel: "Sort out start and end positions" -> [_ _ _ _ _ _ w757 w764 w771 _ w810 _ w831 _ _ _ _ _ _ _ _ _ _ _]
          tunnel: "Check for Start NaNs" -> [w716 _ _ _ w747 w750 _ _ _ w797 _ _ w833 _ _ _ _ _ _ _ _ _ _ _]
          tunnel: [w713 w725 w738 w742 w746 w751 w756 w763 w770 w798 w809 w824 w829 w969 w974 w978 w1018 w1085 w1113 w1118 w1122 w1134 w1138 w1142] -> w694
          tunnel: w693 -> [_ _ _ _ _ _ _ _ _ _ _ _ _ _ _ _ w1024 _ _ _ _ _ _ _]
          frame "Move Traverse Only" {
            w707 = "No Backlash" ("y")
            n265 = Unbundle By Name(w714) -> ("Specific Arguments"=w715:string)
            n266 = call <vilib>:"Trim Whitespace.vi"("string"=w715) -> ("trimmed string"=w709:string)  [unwired: 1 in]
            n267 = Equal?(x=w709, y=w707) -> (x = y?=w712:bool)
            n268 = Empty String/Path?(string/path=w709) -> (empty?=w711:bool)
            n269 = Or(x=w711, y=w712) -> (x .or. y?=w710:bool)
            n270 = case shown="False" w710 {
              tunnel: w709 -> [w720 _]
              tunnel: [w719 ""] -> w708
              tunnel: w707 -> [w718 _]
              frame False {
                n271 = Format Into String(format string="\"%s\" is an Incorrect Specific Argument. It should either be left blank or say \"%s\"\n", w720, w718) -> (resulting string=w719:string)  [unwired: 2 in, 1 out]
              }
              frame True {
              }
            }
            n272 = Bundle By Name(cluster=w714, "Specific Arguments"=w709) -> (w713:T1)
          }
          frame "Set Tunnel Speed Only" {
            w723 = "Do Not Wait" ("y")
            n273 = Unbundle By Name(w725) -> ("Specific Arguments"=w730:string)
            n274 = call <vilib>:"Trim Whitespace.vi"("string"=w730) -> ("trimmed string"=w726:string)  [unwired: 1 in]
            n275 = Equal?(x=w726, y=w723) -> (x = y?=w729:bool)
            n276 = Empty String/Path?(string/path=w726) -> (empty?=w728:bool)
            n277 = Or(x=w728, y=w729) -> (x .or. y?=w727:bool)
            n278 = case shown="False" w727 {
              tunnel: w726 -> [w735 _]
              tunnel: [w734 ""] -> w724
              tunnel: w723 -> [w733 _]
              frame False {
                n279 = Format Into String(format string="\"%s\" is an Incorrect Specific Argument. It should either be left blank or say \"%s\"\n", w735, w733) -> (resulting string=w734:string)  [unwired: 2 in, 1 out]
              }
              frame True {
              }
            }
            n280 = Bundle By Name(cluster=w725, "Specific Arguments"=w726) -> ()  [unwired: 1 out]
          }
          frame "Jump to Fall Back Row" {
          }
          frame "Set Source Only" {
          }
          frame "Set Measurement Conditions" {
          }
          frame "Single Measurement" {
            n281 = Build Array("Averaging:Time:(mins)" ("Label for value"), "Filename:HD:Users" ("Label for value")) -> (w752:string[])
          }
          frame "Vertical Profile" {
            n282 = Build Array("Number:Of:Points" ("Label for value"), "Averaging:Time:(mins)" ("Label for value"), "Filename:HD:Users" ("Label for value")) -> (w759:string[])
          }
          frame "Lateral Profile" {
            n283 = Build Array("Number:Of:Points" ("Label for value"), "Averaging:Time:(mins)" ("Label for value"), "Filename:HD:Users" ("Label for value")) -> (w766:string[])
          }
          frame "Longitudinal Profile" {
            n284 = Build Array("Number:Of:Points" ("Label for value"), "Averaging:Time:(mins)" ("Label for value"), "Filename:HD:Users" ("Label for value")) -> (w773:string[])
          }
          frame "Explore Volume" {
            n285 = Unbundle By Name(w798) -> ("Specific Arguments"=w792:string)
            n286 = Build Array("Averaging:Time:(mins)" ("Label for value"), "Filename:HD:Users" ("Label for value")) -> (w802:string[])
            n287 = call "Get_array_values_fr_String.vi"("String Value"=w792) -> ("Numeric Array"=w793:dbl[], "String array"=w794:string[])
            n288 = Index Array(array=w793) -> (element=w791:dbl)  [unwired: 1 in]
            n289 = Index Array(array=w794, index=1) -> (element=w790:string)
            n290 = To Upper Case(1:w790) -> (0:w778:string)
            n291 = String Subset(string=w778, length (rest)=1 ("length (rest)")) -> (substring=w777:string)  [unwired: 1 in]
            n292 = Greater Than 0?(x=w791) -> (x > 0?=w796:bool)
            n293 = Empty String/Path?(string/path=w790) -> (empty?=w783:bool)
            n294 = Format Into String(format string="\"%s\" is an Incorrect Specific Argument. Please enter the radius of the volume in mm.\n", w792) -> (resulting string=w799:string)  [unwired: 2 in, 1 out]
            n295 = Equal?(x=w777, y="Y") -> (x = y?=w785:bool)
            n296 = Equal?(x=w777, y="X") -> (x = y?=w784:bool)
            n297 = Equal?(x=w777, y="Z") -> (x = y?=w786:bool)
            n298 = Compound Arithmetic op=OR(w783, w784, w785, w786) -> (w782:bool)
            n299 = Select(t="", s=w796, f=w799) -> (s? t:f=w780:string)
            n300 = case shown="False" w782 {
              tunnel: [w805 w808] -> w781
              tunnel: w780 -> [w806 w808]
              frame False {
                n301 = Concatenate Strings(w806, "Second Specific Argument should be the axis that should remain fixed, eg X_Fixed or Y_Fixed" ("string")) -> (w805:string)
              }
              frame True {
              }
            }
          }
          frame "Multi-Axis Profile" {
            n302 = Unbundle By Name(w809) -> ("Spacing"=w812:T2)
            n303 = Build Array("Number:Of:Points" ("Label for value"), "Averaging:Time:(mins)" ("Label for value"), "Filename:HD:Users" ("Label for value")) -> (w814:string[])
            n304 = case shown="\"Linear\", Default" w812 {
              tunnel: ["" "You are not allowed to specify gaussian spacing for a Multi-Axis profile.\n" "You are not allowed to specify Log spacing for a Multi-Axis profile.\n" "\"N/A\" is not a valid point spacing.\n"] -> w811
              frame "Linear", Default {
              }
              frame "Gauss" {
              }
              frame "Log" {
              }
              frame "N/A" {
              }
            }
          }
          frame "Traverse 3D Volume" {
            n305 = Build Array("Number:Of:Points" ("Label for value"), "Averaging:Time:(mins)" ("Label for value"), "Filename:HD:Users" ("Label for value")) -> (w825:string[])
          }
          frame "Auto Calibrate" {
            n306 = stacked-sequence {
              seq-local: [w838 _ _ _ _ _] -> [_ _ _ _ _ w958]
              seq-local: [w837 _ _ _ _ _] -> [_ w868 w879 _ w946 _]
              seq-local: [w836 _ _ _ _ _] -> [_ w867 w882 w909 w948 _]
              seq-local: [_ w866 _ _ _ _] -> [_ _ _ _ _ w957]
              seq-local: [_ _ _ w911 _ _] -> [_ _ _ _ _ w956]
              seq-local: [_ _ _ _ w939 _] -> [_ _ _ _ _ w954]
              seq-local: [_ _ w880 _ _ _] -> [_ _ _ _ _ w953]
              tunnel: [w847 _ _ _ _ _] -> w834
              tunnel: w833 -> [w846 _ _ _ _ _]
              tunnel: [w845 _ _ _ _ _] -> w832
              tunnel: w831 -> [w844 _ _ _ _ _]
              tunnel: w830 -> [w843 _ _ w910 w941 _]
              tunnel: [_ _ _ w908 _ _] -> w829
              tunnel: [_ _ _ _ _ w955] -> w828
              frame #0 {
                n307 = Unbundle By Name(w843) -> ("Specific Arguments"=w840:string)
                n308 = call "Get_array_values_fr_String.vi"("String Value"=w840) -> ("Numeric Array"=w837:dbl[], "String array"=w841:string[])
                n309 = Build Array("Tunnel Speed", "Traverse Position", "Concentration", "ESC RPM") -> (w850:string[])
                n310 = Index Array(array=w841, index=0 ("Index")) -> (element=w839:string)
                n311 = Build Array("Averaging:Time:(mins)" ("Label for value")) -> (w847:string[])
                n312 = Search 1D Array(1D array=w850, element=w839) -> (index of element=w836:i32)  [unwired: 1 out]
                n313 = case shown="0, Default" w836 {
                  tunnel: [w864 w865] -> w845
                  tunnel: w846 -> [w864 _]
                  tunnel: w844 -> [_ w865]
                  frame 0, Default {
                  }
                  frame 1 {
                  }
                }
                n314 = Greater Or Equal To 0?(x=w836) -> (x >= 0?=w848:bool)
                n315 = case shown="False" w848 {
                  tunnel: w850 -> [w855 _]
                  tunnel: [w854 ""] -> w838
                  frame False {
                    n316 = for {
                      shift-right: [w860] -> w857
                      shift-left: "Incorrect Specific Argument. The options are: " -> [w861]
                      tunnel: w855 -> [w862] mode=indexing
                      w859 = "  " ("Substring")
                      n317 = Concatenate Strings(w861, w859, w862, w859) -> (w860:string)
                    }
                    n318 = Concatenate Strings(w857, "\r\n") -> (w854:string)
                  }
                  frame True {
                  }
                }
              }
              frame #1 {
                n319 = Equal To 0?(x=w867) -> (x = 0?=w872:bool)
                n320 = Array Size(array=w868) -> (size(s)=w875:i32)
                n321 = Less?(x=w875, y=3) -> (x < y?=w871:bool)
                n322 = Compound Arithmetic op=AND(w871, w872) -> (w870:bool)
                n323 = Select(t="You need to enter the desired tunnel speeds in the \"Specfic Arguments\" Box   eg.  Tunnel Speed;1;2;3;4\n", s=w870, f="") -> (s? t:f=w866:string)
              }
              frame #2 {
                n324 = Array Subset(array=w879, index=1) -> (w876:dbl[])  [unwired: 1 in]
                n325 = Array Size(array=w876) -> (size(s)=w885:i32)
                n326 = Equal?(x=w882, y=3) -> (x = y?=w877:bool)
                n327 = Less?(x=w885, y=3) -> (x < y?=w883:bool)
                n328 = case shown="True" w877 {
                  tunnel: w883 -> [_ w894]
                  tunnel: ["" w890] -> w880
                  tunnel: w876 -> [_ w893]
                  frame False {
                  }
                  frame True {
                    n329 = for {
                      tunnel: w893 -> [w907] mode=indexing
                      tunnel: [w906] -> w892 mode=indexing
                      tunnel: [w905] -> w888
                      tunnel: [w904] -> w887
                      w904 = 100.0 ("upper limit")
                      w905 = 0.0 ("lower limit")
                      n330 = In Range and Coerce(upper limit=w904, x=w907, lower limit=w905) -> (In Range?=w906:bool)  [unwired: 1 out]
                    }
                    n331 = And Array Elements(Boolean array=w892) -> (logical AND=w891:bool)
                    n332 = Select(t="You need to enter the desired  PWMs in the \"Specfic Arguments\" Box   eg.  ESC RPM; 20; 30;40;", s=w894, f="") -> (s? t:f=w889:string)
                    n333 = case shown="False" w891 {
                      tunnel: [w902 w903] -> w890
                      tunnel: w889 -> [w901 w903]
                      tunnel: w888 -> [w900 _]
                      tunnel: w887 -> [w899 _]
                      frame False {
                        n334 = Format Into String(format string="PWM should be in the range %.0f to %.0f\n", w900, w899) -> (resulting string=w897:string)  [unwired: 2 in, 1 out]
                        n335 = Concatenate Strings(w897, w901) -> (w902:string)
                      }
                      frame True {
                      }
                    }
                  }
                }
              }
              frame #3 {
                n336 = global read "Trav_pos_global.vi" "Work in Tunnel Coordinates?"() -> (w922:T7)
                n337 = Unbundle By Name(w910) -> ("Filename"=w915:path)
                n338 = call "Current_Filepath.vi"("Short_Name"="Cal" ("Data Type"), "Filename in"=w915, "Data Type"="Calibrations") -> ("Filename Out"=w913:path)  [unwired: 1 in, 1 out]
                n339 = Equal?(x=w922, y=Tunnel_Coordinates."Work in Model Coordinates" ("Work in Tunnel Coordinates?")) -> (x = y?=w917:bool)
                n340 = Equal?(x=2, y=w909) -> (x = y?=w919:bool)
                n341 = And(x=w917, y=w919) -> (x .and. y?=w918:bool)
                n342 = case shown="False" w918 {
                  tunnel: [w926 w931] -> w914
                  tunnel: w910 -> [w926 w927]
                  frame False {
                  }
                  frame True {
                    n343 = global read "Extra_Commands_Global.vi" "Work in Tunnel Coordinates"() -> (w929:string)
                    n344 = Unbundle By Name(w927) -> ("Extra Commands"=w928:string)
                    n345 = call "Extra_Commands.vi"("String to Search"=w928, "Command"=w929) -> ("Command Found"=w930:bool)  [unwired: 1 in, 4 out]
                    n346 = case shown="False" w930 {
                      tunnel: [w937 w938] -> w931
                      tunnel: w929 -> [w936 _]
                      tunnel: w928 -> [w935 _]
                      tunnel: w927 -> [w933 w938]
                      frame False {
                        n347 = Concatenate Strings(w936, "  " ("string"), w935) -> (w934:string)
                        n348 = Bundle By Name(cluster=w933, "Extra Commands"=w934) -> (w937:T1)
                      }
                      frame True {
                      }
                    }
                  }
                }
                n349 = call "Does_file_exist_(simple).vi"("Pathname"=w913) -> ("exists?"=w925:bool)
                n350 = Select(t="", s=w925, f="The calibration file cannot be found.\n") -> (s? t:f=w911:string)
                n351 = Bundle By Name(cluster=w914, "Filename"=w913) -> (w908:T1)
              }
              frame #4 {
                n352 = Equal?(x=2, y=w948) -> (x = y?=w943:bool)
                n353 = Array Size(array=w946) -> (size(s)=w940:i32)
                n354 = Greater?(x=w940, y=1) -> (0:w944:bool)
                n355 = And(x=w944, y=w943) -> (x .and. y?=w942:bool)
                n356 = case shown="True" w942 {
                  tunnel: w941 -> [_ w952]
                  tunnel: w940 -> [_ _]
                  tunnel: ["" w950] -> w939
                  frame False {
                  }
                  frame True {
                    n357 = Unbundle By Name(w952) -> ("Specific Arguments"=w951:string)
                    n358 = call "Read_FFID_Auto_Calib_Setup.vi"("Specific Argument"=w951) -> ("Error String"=w950:string)  [unwired: 4 out]
                  }
                }
              }
              frame #5 {
                n359 = Concatenate Strings(w958, w957, w953, w956, w954) -> (w955:string)
              }
            }
          }
          frame "Meas Fast FID Bkgnd" {
            n360 = Unbundle By Name(w969) -> ("Specific Arguments"=w964:string)
            n361 = call "Get_array_values_fr_String.vi"("String Value"=w964) -> ("String array"=w963:string[])  [unwired: 1 out]
            n362 = Index Array(array=w963, index=0) -> (element=w961:string)
            n363 = Empty String/Path?(string/path=w961) -> (empty?=w967:bool)
            n364 = Build Array("Averaging:Time:(mins)" ("Label for value")) -> (w971:string[])
            n365 = Equal?(x=w961, y="Use Source Divertor Valve") -> (x = y?=w960:bool)
            n366 = Or(x=w967, y=w960) -> (x .or. y?=w966:bool)
            n367 = case shown="False" w966 {
              tunnel: ["Specific Argument should either be blank or\nUse Source Divertor Valve ; (wait time in seconds optional)" ""] -> w965
              frame False {
              }
              frame True {
              }
            }
          }
          frame "Check Beam Power" {
          }
          frame "Scanning Valve Measurement" {
            w991 = ext -0.5  # lo
            w992 = ext 47.5  # hi
            n368 = Unbundle By Name(w978) -> ("Specific Arguments"=w988:string)
            n369 = call "Get_array_values_fr_String.vi"("String Value"=w988) -> ("Numeric Array"=w987:dbl[], "String array"=w983:string[])
            n370 = Build Array("Averaging:Time:(mins)" ("Label for value"), "Filename:HD:Users" ("Label for value")) -> (w995:string[])
            n371 = Index Array(array=w983, index=0) -> (element=w982:string)
            n372 = Empty String/Path?(string/path=w982) -> (empty?=w980:bool)
            n373 = Index Array(array=w987, index=0) -> (element=w985:dbl)
            n374 = In Range and Coerce(upper limit=w992, x=w985, lower limit=w991) -> (In Range?=w981:bool)  [unwired: 1 out]
            n375 = Compound Arithmetic op=AND(invert w980, w981) -> (w979:bool)
            n376 = Select(t="", s=w979, f="Enter the scanning valve port number between 0 and 47 in the specific arguments box.\n") -> (s? t:f=w990:string)
          }
          frame "Set ADAM Ch" {
            w998 = "EnFlo_Tunnel:Heater:Enable"
            n377 = Unbundle By Name(w1019) -> ("Specific Arguments"=w1026:string, "Extra Commands"=w1015:string)
            n378 = global read "Trav_pos_global.vi" "Multi_Run_Prog_Start_Time"() -> (w1004:dbl)
            n379 = while {
              shift-right: [w1074] -> w1025
              shift-left: _ -> [w1070]
              shift-right: [w1068] -> _
              shift-left: _ -> [w1067]
              tunnel: w1004 -> [w1068]
              stop <- TRUE stop-if-true
              n380 = Array Size(array=w1070) -> (size(s)=w1073:i32)
              n381 = Not Equal?(x=w1067, y=w1068) -> (x != y?=w1066:bool)
              n382 = Equal To 0?(x=w1073) -> (x = 0?=w1072:bool)
              n383 = Or(x=w1072, y=w1066) -> (x .or. y?=w1071:bool)
              n384 = case shown="True" w1071 {
                tunnel: [w1075 w1076] -> w1074
                tunnel: w1070 -> [w1075 _]
                frame False {
                }
                frame True {
                  n385 = call "Get_ADAM_Ch_names_client.vi"("Channel names set"=Channel_names."Active + Off") -> ("Ch names"=w1076:string[])
                }
              }
            }
            n386 = call "Get_array_values_fr_String.vi"("String Value"=w1015) -> ("Numeric Array"=w999:dbl[])  [unwired: 1 out]
            n387 = call "Get_array_values_fr_String.vi"("String Value"=w1026) -> ("String array"=w1003:string[])  [unwired: 1 out]
            n388 = for {
              tunnel: w1025 -> [w1048]
              tunnel: w1003 -> [w1047] mode=indexing
              tunnel: w999 -> [w1043]
              tunnel: [w1045] -> w1014 mode=indexing
              tunnel: [w1044] -> w1013 mode=indexing
              i -> [w1042]
              n389 = Index Array(array=w1043, index=w1042) -> (element=w1046:dbl)
              n390 = Search 1D Array(1D array=w1048, element=w1047) -> (index of element=w1049:i32)  [unwired: 1 out]
              n391 = Not A Number/Path/Refnum?(number/path/refnum=w1046) -> (NaN/Path/Refnum?=w1044:bool)
              n392 = Greater Or Equal To 0?(x=w1049) -> (x >= 0?=w1045:bool)
            }
            n393 = Array Size(array=w1003) -> (size(s)=w1008:i32)
            n394 = Array Size(array=w999) -> (size(s)=w1012:i32)
            n395 = Not Equal?(x=w1008, y=w1012) -> (x != y?=w1010:bool)
            n396 = Search 1D Array(1D array=w1003, element=w998) -> (index of element=w1000:i32)  [unwired: 1 in]
            n397 = Greater Than 0?(x=w1008) -> (x > 0?=w1006:bool)
            n398 = Or Array Elements(Boolean array=w1013) -> (logical OR=w1011:bool)
            n399 = And Array Elements(Boolean array=w1014) -> (logical AND=w1007:bool)
            n400 = Or(x=w1010, y=w1011) -> (x .or. y?=w1009:bool)
            n401 = Select(t="You have not specified a Value to Set the ADAM channel to.\nPlease give the values separated by ; in the Extra Commands string", s=w1009, f="") -> (s? t:f=w1001:string)
            n402 = case shown="Default" w1000 {
              tunnel: [w1030 w1041] -> w1002
              tunnel: w1001 -> [w1029 w1041]
              tunnel: w1000 -> [w1035 _]
              tunnel: w999 -> [w1034 _]
              tunnel: w998 -> [w1028 _]
              frame Default {
                n403 = Index Array(array=w1034, index=w1035) -> (element=w1033:dbl)
                n404 = Greater?(x=w1033, y=0.5) -> (0:w1031:bool)
                n405 = case shown="True" w1031 {
                  tunnel: [w1036 w1037] -> w1030
                  tunnel: w1029 -> [w1036 w1038]
                  tunnel: w1028 -> [_ w1040]
                  frame False {
                  }
                  frame True {
                    n406 = Format Into String(format string="You are not allowed to programmatically turn on %s.", initial string=w1038, w1040) -> (resulting string=w1037:string)  [unwired: 1 in, 1 out]
                  }
                }
              }
              frame -1 {
              }
            }
            n407 = And(x=w1006, y=w1007) -> (x .and. y?=w1005:bool)
            n408 = case shown="True" w1005 {
              tunnel: w1025 -> [w1060 _]
              tunnel: w1003 -> [w1052 w1062]
              tunnel: w1024 -> [w1058 _]
              tunnel: [w1056 FALSE ("Cancel")] -> w1023
              tunnel: w1019 -> [w1054 w1064]
              tunnel: [w1053 w1063] -> w1018
              frame False {
                n409 = Format Into String(format string="Please Select the ADAM Channels that you want to set in row %d", w1058) -> (resulting string=w1057:string)  [unwired: 2 in, 1 out]
                n410 = call "Select_Strings.vi"("Available Ch names"=w1060, "Message"=w1057, "Selector mode"=T8."One or more", "Desired Ch names (in)"=w1052) -> ("Cancel"=w1056:bool, "Selected Channel Names"=w1051:string[])  [unwired: 1 in, 2 out]
                n411 = call "Put_Array_into_String.vi"("String array"=w1051) -> ("String Value"=w1050:string)
                n412 = Bundle By Name(cluster=w1054, "Specific Arguments"=w1050) -> (w1053:T1)
              }
              frame True {
                n413 = call "Put_Array_into_String.vi"("String array"=w1062) -> ("String Value"=w1061:string)
                n414 = Bundle By Name(cluster=w1064, "Specific Arguments"=w1061) -> (w1063:T1)
              }
            }
            n415 = Select(t="Close Front Panel", s=w1023, f=w1021) -> (s? t:f=w1022:string)
          }
          frame "Run VI Named:" {
            w1090 = "Run_VI_Named_specific.vi"
            n416 = Unbundle By Name(w1085) -> ("Specific Arguments"=w1093:string)
            n417 = global read "Constants_global.vi" "Run VI Folder"() -> (w1091:path)
            n418 = Match Pattern(string=w1093, regular expression=";") -> (before substring=w1094:string)  [unwired: 4 out]
            n419 = call <vilib>:"Trim Whitespace.vi"("string"=w1094) -> ("trimmed string"=w1086:string)  [unwired: 1 in]
            n420 = call "Run_VI_Named_specific.vi"("Run VI Named String"=w1086, "Earlier Filenames"="Earlier Filenames", "Multi Run Row"=w1085) -> ("Checks"=w1080:string[], "Error String"=w1079:string, "Check for start NaNs?"=w1084:bool)  [unwired: 6 out]
            n421 = Select(t="Check for Start NaNs" ("Label for value"), s=w1084, f=w1082) -> (s? t:f=w1081:string)
            n422 = Build Path(base path=w1091, name or relative path=w1086) -> (appended path=w1097:path)
            n423 = Not Equal?(x=w1086, y=w1090) -> (x != y?=w1089:bool)
            n424 = call "Does_file_exist_(simple).vi"("Pathname"=w1097) -> ("exists?"=w1088:bool)
            n425 = And(x=w1088, y=w1089) -> (x .and. y?=w1087:bool)
            n426 = case shown="False" w1087 {
              tunnel: [w1104 ""] -> w1092
              tunnel: w1091 -> [w1100 _]
              tunnel: w1090 -> [w1098 _]
              frame False {
                w1102 = "\r\n"
                n427 = Build Array(w1098) -> (w1099:string[])
                n428 = call "List_files_in_order_of_age.vi"("Files to Hide"=w1099, "Folder"=w1100) -> ("file names"=w1101:string[])  [unwired: 9 in]
                n429 = for {
                  shift-right: [w1108] -> w1105
                  shift-left: "Cannot find the VI to run. Specific Argument options are:" -> [w1109]
                  tunnel: w1101 -> [w1110] mode=indexing
                  w1107 = "  " ("Substring")
                  n430 = Concatenate Strings(w1109, w1107, w1110, w1107) -> (w1108:string)
                }
                n431 = Concatenate Strings(w1105, w1102, "Please place one of these strings in the \"Specific Argument\" field.", w1102) -> (w1104:string)
              }
              frame True {
              }
            }
            n432 = Concatenate Strings(w1079, w1092) -> (w1096:string)
          }
          frame "Wait (minutes)" {
            n433 = Unbundle By Name(w1113) -> ("Specific Arguments"=w1114:string)
            n434 = call "Wait_Case_Arg.vi"("Specific Argument"=w1114) -> ("Error Comments"=w1115:string)  [unwired: 1 in, 4 out]
          }
          frame "Send Message" {
          }
          frame "Synchronize With:" {
            n435 = local read "Current Sync Number"() -> (w1123:i32)
            n436 = call "Synchronize_Prog_Arg.vi"("Execution Row"=w1122) -> ("Error Comments"=w1125:string, "Sync No"=w1131:i32)  [unwired: 3 out]
            n437 = Format Into String(format string="This should be Synchroisation number %d.\n" ("Format String"), w1123) -> (resulting string=w1128:string)  [unwired: 2 in, 1 out]
            n438 = Equal?(x=w1131, y=w1123) -> (x = y?=w1130:bool)
            n439 = Select(t="", s=w1130, f=w1128) -> (s? t:f=w1126:string)
            n440 = Concatenate Strings(w1126, w1125) -> (w1124:string)
          }
          frame "Fall Back to this Row" {
          }
          frame "Turn Off Row Repeating" {
          }
          frame "Blank Row" {
            n441 = Unbundle By Name(w1144) -> ("Comments"=w1150:string)
            n442 = Match Pattern(string=w1150, regular expression="(No Match Info)") -> (before substring=w1143:string, after substring=w1147:string)  [unwired: 3 out]
            n443 = Empty String/Path?(string/path=w1147) -> (empty?=w1148:bool)
            n444 = Bundle By Name(cluster=w1144, "Comments"=w1143) -> (w1142:T1)
            n445 = Select(t=w1147, s=w1148, f="The Row Type Selector \"%s\" was not matched. Please select the desired type.\n") -> (s? t:f=w1146:string)
          }
        }
        "Checks" <- w701
        n446 = Concatenate Strings(w704, w705) -> (w703:string)
      }
      frame "Sort out start and end positions" {
        n447 = Unbundle By Name(w1158) -> ("Start X"=w1170:sgl, "Start Y"=w1169:sgl, "Start Z"=w1168:sgl, "End X"=w1167:sgl, "End Y"=w1166:sgl, "End Z"=w1165:sgl, "Extra Commands"=w1154:string)
        n448 = call "Which_Trav_Setup.vi"("Extra Command String"=w1154) -> ("Traverse Setups"=w1152:string[])  [unwired: 2 out]
        n449 = Build Array(w1170, w1169, w1168) -> (w1161:sgl[])
        n450 = Build Array(w1167, w1166, w1165) -> (w1160:sgl[])
        n451 = Index Array(array=w1152) -> (element=w1153:string)  [unwired: 1 in]
        n452 = call "Rig_Pict_Display_Pref.vi"("Traverse Name"=w1153) -> ("Which Axis is vertical?"=w1164:enum16{"X Axis", "Y Axis", "Z Axis"})  [unwired: 7 out]
        n453 = case shown="\"Multi-Axis Profile\", Default" w1159 {
          tunnel: [w1210 FALSE w1226 w1239 FALSE] -> w1173
          tunnel: [w1209 FALSE w1225 w1238 FALSE] -> w1172
          tunnel: [w1208 FALSE w1224 w1237 FALSE] -> w1171
          tunnel: w1164 -> [w1207 _ w1223 w1236 _]
          frame "Vertical Profile" {
            n454 = case shown="\"Z Axis\"" w1207 {
              tunnel: [FALSE TRUE TRUE] -> w1210
              tunnel: [TRUE FALSE TRUE] -> w1209
              tunnel: [TRUE TRUE FALSE] -> w1208
              frame "X Axis" {
              }
              frame "Y Axis" {
              }
              frame "Z Axis" {
              }
            }
          }
          frame "Auto Calibrate" {
          }
          frame "Lateral Profile" {
            n455 = case shown="\"Y Axis\"" w1223 {
              tunnel: [TRUE TRUE TRUE] -> w1226
              tunnel: [TRUE TRUE FALSE] -> w1225
              tunnel: [FALSE FALSE TRUE] -> w1224
              frame "X Axis" {
              }
              frame "Y Axis" {
              }
              frame "Z Axis" {
              }
            }
          }
          frame "Longitudinal Profile" {
            n456 = case shown="\"Y Axis\"" w1236 {
              tunnel: [FALSE FALSE FALSE] -> w1239
              tunnel: [TRUE TRUE TRUE] -> w1238
              tunnel: [TRUE TRUE TRUE] -> w1237
              frame "X Axis" {
              }
              frame "Y Axis" {
              }
              frame "Z Axis" {
              }
            }
          }
          frame "Multi-Axis Profile", Default {
          }
        }
        n457 = Build Array(w1173, w1172, w1171) -> (w1162:bool[])
        "Fixed Axis" <- w1162
        n458 = for {
          tunnel: w1162 -> [w1180] mode=indexing
          tunnel: w1161 -> [w1179] mode=indexing
          tunnel: w1160 -> [w1178] mode=indexing
          shift-right: [w1175] -> w1157
          shift-left: w1158 -> [w1176]
          i -> [w1177]
          n459 = case shown="True" w1180 {
            tunnel: w1179 -> [_ w1186]
            tunnel: w1178 -> [_ w1185]
            tunnel: w1177 -> [_ w1184]
            tunnel: w1176 -> [w1181 w1183]
            tunnel: [w1181 w1182] -> w1175
            frame False {
            }
            frame True {
              n460 = Not A Number/Path/Refnum?(number/path/refnum=w1186) -> (NaN/Path/Refnum?=w1187:bool)
              n461 = Not A Number/Path/Refnum?(number/path/refnum=w1185) -> (NaN/Path/Refnum?=w1189:bool)
              n462 = Exclusive Or(1:w1189, 2:w1187) -> (0:w1188:bool)
              n463 = case shown="True" w1188 {
                tunnel: w1187 -> [_ w1197]
                tunnel: w1186 -> [_ w1196]
                tunnel: w1185 -> [_ w1195]
                tunnel: w1184 -> [_ w1194]
                tunnel: w1183 -> [w1190 w1193]
                tunnel: [w1190 w1192] -> w1182
                frame False {
                }
                frame True {
                  n464 = Select(t=w1195, s=w1197, f=w1196) -> (s? t:f=w1191:sgl)
                  n465 = case shown="2" w1194 {
                    tunnel: w1193 -> [w1200 w1203 w1206]
                    tunnel: [w1199 w1202 w1205] -> w1192
                    tunnel: w1191 -> [w1198 w1201 w1204]
                    frame 0, Default {
                      n466 = Bundle By Name(cluster=w1200, "Start X"=w1198, "End X"=w1198) -> (w1199:T1)
                    }
                    frame 1 {
                      n467 = Bundle By Name(cluster=w1203, "Start Y"=w1201, "End Y"=w1201) -> (w1202:T1)
                    }
                    frame 2 {
                      n468 = Bundle By Name(cluster=w1206, "Start Z"=w1204, "End Z"=w1204) -> (w1205:T1)
                    }
                  }
                }
              }
            }
          }
        }
      }
      frame "Check for position NaNs" {
        n469 = global read "Extra_Commands_Global.vi" "Skip Traverse Position Demand"() -> (w1257:string)
        n470 = Unbundle By Name(w1259) -> ("Extra Commands"=w1256:string, "Start X"=w1268:sgl, "Start Y"=w1266:sgl, "Start Z"=w1267:sgl, "End X"=w1265:sgl, "End Y"=w1264:sgl, "End Z"=w1263:sgl)
        n471 = call "Extra_Commands.vi"("String to Search"=w1256, "Command"=w1257) -> ("Command Found"=w1254:bool)  [unwired: 1 in, 4 out]
        n472 = case shown="False" w1254 {
          tunnel: w1268 -> [w1283 _]
          tunnel: w1267 -> [w1282 _]
          tunnel: w1266 -> [w1281 _]
          tunnel: w1265 -> [w1280 _]
          tunnel: w1264 -> [w1279 _]
          tunnel: w1263 -> [w1278 _]
          tunnel: [w1274 w1284] -> w1262
          tunnel: [w1273 TRUE] -> w1261
          tunnel: "" -> [w1272 w1284]
          frame False {
            n473 = Build Array(w1283, w1281, w1282, w1280, w1279, w1278) -> (w1277:sgl[])
            n474 = Not A Number/Path/Refnum?(number/path/refnum=w1277) -> (NaN/Path/Refnum?=w1276:bool[])
            n475 = Or Array Elements(Boolean array=w1276) -> (logical OR=w1273:bool)
            n476 = Select(t="Some of the Start and End positions are NaN.\n" ("f"), s=w1273, f=w1272) -> (s? t:f=w1274:string)
          }
          frame True {
          }
        }
        n477 = Select(t="Check source details", s=w1261, f="Check profile rows") -> (s? t:f=w1260:string)
        n478 = Concatenate Strings(w1270, w1262) -> (w1269:string)
      }
      frame "Check for Start NaNs" {
        n479 = Unbundle By Name(w1291) -> ("Extra Commands"=w1287:string, "Start X"=w1296:sgl, "Start Y"=w1294:sgl, "Start Z"=w1295:sgl)
        n480 = global read "Extra_Commands_Global.vi" "Skip Traverse Position Demand"() -> (w1288:string)
        n481 = call "Extra_Commands.vi"("String to Search"=w1287, "Command"=w1288) -> ("Command Found"=w1286:bool)  [unwired: 1 in, 4 out]
        n482 = case shown="False" w1286 {
          tunnel: w1296 -> [w1311 _]
          tunnel: w1295 -> [w1310 _]
          tunnel: w1294 -> [w1309 _]
          tunnel: "" -> [w1307 w1312]
          tunnel: [w1305 w1312] -> w1292
          frame False {
            n483 = Build Array(w1311, w1309, w1310) -> (w1308:sgl[])
            n484 = Not A Number/Path/Refnum?(number/path/refnum=w1308) -> (NaN/Path/Refnum?=w1304:bool[])
            n485 = Boolean To (0,1)(Boolean=w1304) -> (0, 1=w1303:i16[])
            n486 = Add Array Elements(numeric array=w1303) -> (sum=w1302:i16)
            n487 = Greater?(x=w1302, y=i16 2) -> (0:w1300:bool)
            n488 = Select(t="Only up to two of the Start coordinates can be  NaN.\n" ("f"), s=w1300, f=w1307) -> (s? t:f=w1305:string)
          }
          frame True {
          }
        }
        n489 = Concatenate Strings(w1298, w1292) -> (w1297:string)
      }
      frame "Check profile rows" {
        n490 = Unbundle By Name(w1322) -> ("Start X"=w1343:sgl, "Start Y"=w1342:sgl, "Start Z"=w1341:sgl, "End X"=w1340:sgl, "End Y"=w1339:sgl, "End Z"=w1338:sgl, "Specific Arguments"=w1332:string, "Spacing"=w1327:T2)
        n491 = local read "Fixed Axis"() -> (w1326:bool[])
        n492 = Build Array(w1343, w1342, w1341) -> (w1324:sgl[])
        n493 = Build Array(w1340, w1339, w1338) -> (w1325:sgl[])
        n494 = case shown="\"Gauss\"" w1327 {
          tunnel: w1332 -> [_ _ _ _ _]
          tunnel: ["" w1351 "\"N/A\" is not a valid point spacing.\n" "" ""] -> w1331
          tunnel: w1326 -> [_ w1349 _ _ _]
          tunnel: w1325 -> [_ w1356 _ _ _]
          tunnel: w1324 -> [_ w1355 _ _ _]
          frame "Linear" {
          }
          frame "Log" {
            n495 = for {
              tunnel: w1356 -> [w1360] mode=indexing
              tunnel: w1355 -> [w1359] mode=indexing
              tunnel: [w1358] -> w1354 mode=indexing
              tunnel: w1349 -> [w1357] mode=indexing
              n496 = case shown="False" w1357 {
                tunnel: w1360 -> [w1366 _]
                tunnel: w1359 -> [w1365 _]
                tunnel: [w1361 FALSE] -> w1358
                frame False {
                  w1364 = 0.001 ("y")
                  n497 = Less?(x=w1366, y=w1364) -> (x < y?=w1362:bool)
                  n498 = Less?(x=w1365, y=w1364) -> (x < y?=w1363:bool)
                  n499 = Or(x=w1362, y=w1363) -> (x .or. y?=w1361:bool)
                }
                frame True {
                }
              }
            }
            n500 = Or Array Elements(Boolean array=w1354) -> (logical OR=w1353:bool)
            n501 = Select(t="For log spacing, Start & End positions must be greater than 0.0001.", s=w1353, f="") -> (s? t:f=w1351:string)
          }
          frame "N/A" {
          }
          frame "Gauss" {
          }
          frame "Specified" {
          }
        }
        n502 = for {
          tunnel: w1326 -> [w1376] mode=indexing
          tunnel: w1324 -> [w1375] mode=indexing
          tunnel: w1325 -> [w1374] mode=indexing
          tunnel: [w1373] -> w1337 mode=indexing
          shift-right: [w1371] -> w1317
          shift-left: bool[] [] -> [w1372]
          n503 = case shown="False" w1376 {
            tunnel: w1375 -> [w1380 w1386]
            tunnel: w1374 -> [w1381 w1385]
            tunnel: [TRUE w1384] -> w1373
            tunnel: w1372 -> [w1378 w1383]
            tunnel: [w1377 w1383] -> w1371
            frame False {
              n504 = Not Equal?(x=w1380, y=w1381) -> (x != y?=w1379:bool)
              n505 = Build Array (concatenate)(w1378, w1379) -> (w1377:bool[])
            }
            frame True {
              n506 = Equal?(x=w1386, y=w1385) -> (x = y?=w1384:bool)
            }
          }
        }
        n507 = Array Size(array=w1317) -> (size(s)=w1316:i32)
        n508 = And Array Elements(Boolean array=w1337) -> (logical AND=w1336:bool)
        n509 = Or Array Elements(Boolean array=w1317) -> (logical OR=w1314:bool)
        n510 = Not Equal To 0?(x=w1316) -> (x != 0?=w1315:bool)
        n511 = And(x=w1314, y=w1315) -> (x .and. y?=w1313:bool)
        n512 = call "Create_Pos_array.vi"("Traverse line"=w1322) -> ("Traverse line Out"=w1321:T1, "Error Messages"=w1320:string)  [unwired: 7 out]
        n513 = Select(t="", s=w1336, f="This profile moves more than one axis.\n") -> (s? t:f=w1333:string)
        n514 = Select(t="", s=w1313, f="The start and end points are the same for this profile.\n") -> (s? t:f=w1329:string)
        n515 = Concatenate Strings(w1320, w1329, w1333, w1331) -> (w1346:string)
        n516 = Concatenate Strings(w1345, w1346) -> (w1344:string)
      }
      frame "Check source details" {
        n517 = Unbundle By Name(w1395) -> ("Carrier_1 Q (l/min)"=w1389:dbl, "Carrier_2 Q (l/min)"=w1388:dbl)  [unwired: 1 out]
        n518 = Add(x=w1389, y=w1388) -> (x+y=w1387:dbl)
        n519 = Greater Than 0?(x=w1387) -> (x > 0?=w1393:bool)
        n520 = Select(t="Check source detail 2", s=w1393, f="check entered filename etc") -> (s? t:f=w1391:string)
      }
      frame "Check source detail 2" {
        n521 = global read "Preference_global.vi" "Site Specific String (Blank if Surrey)"() -> (w1398:string)
        n522 = Unbundle By Name(w1403) -> ("Trace Gas Concentration (%)"=w1399:dbl)
        n523 = case shown="\"\", Default" w1398 {
          tunnel: ["" ("f") w1413] -> w1400
          tunnel: w1399 -> [_ w1412]
          frame "CPP" {
          }
          frame "", Default {
            n524 = Equal?(x=w1412, y=100.0) -> (x = y?=w1410:bool)
            n525 = In Range and Coerce(upper limit=ext 2.1099999999999999999 ("hi"), x=w1412, lower limit=ext 0.0 ("lo")) -> (In Range?=w1409:bool)  [unwired: 1 out]
            n526 = Or(x=w1410, y=w1409) -> (x .or. y?=w1408:bool)
            n527 = Select(t="", s=w1408, f="The Trace Gas Concentration must be within the range of 0 to 2.1%  or equal 100%.\n") -> (s? t:f=w1413:string)
          }
        }
        n528 = Concatenate Strings(w1405, w1400) -> (w1404:string)
      }
      frame "check entered filename etc" {
        n529 = local read "Checks"() -> (w1429:string[])
        n530 = for {
          tunnel: w1429 -> [w1436] mode=indexing
          tunnel: [w1441] -> w1430 mode=indexing
          tunnel: w1426 -> [w1440]
          shift-right: [w1438] -> w1420
          shift-left: w1421 -> [w1439]
          tunnel: [w1437] -> w1419 mode=indexing
          n531 = case shown="\"Averaging:Time:(mins)\"" w1436 {
            tunnel: w1439 -> [w1442 w1455 w1480 w1492]
            tunnel: [w1445 w1458 w1486 w1488] -> w1441
            tunnel: w1440 -> [_ _ _ _]
            tunnel: [w1442 w1455 w1479 w1492] -> w1438
            tunnel: [TRUE ("cancelled") TRUE ("cancelled") w1474 TRUE ("cancelled")] -> w1437
            tunnel: w1436 -> [_ _ _ w1490]
            frame "Number:Of:Points" {
              n532 = Unbundle By Name(w1442) -> ("nPoints"=w1447:i32, "Spacing"=w1443:T2)
              n533 = case shown="Default" w1443 {
                tunnel: [TRUE w1452] -> w1449
                tunnel: w1447 -> [_ w1451]
                frame "Specified" {
                }
                frame Default {
                  n534 = Greater?(x=w1451, y=0) -> (0:w1452:bool)
                }
              }
              n535 = Select(t="", s=w1449, f="For a profile the number of points should be more than 0.\n" ("Format String")) -> (s? t:f=w1445:string)
            }
            frame "Averaging:Time:(mins)" {
              n536 = Unbundle By Name(w1455) -> ("Averaging time (mins)"=w1457:dbl)
              n537 = Greater Than 0?(x=w1457) -> (x > 0?=w1456:bool)
              n538 = Select(t="", s=w1456, f="The averaging time should be greater than zero.\n" ("Format String")) -> (s? t:f=w1458:string)
            }
            frame "Filename:HD:Users" {
              w1487 = FALSE  # Show Error handler
              n539 = Unbundle By Name(w1480) -> ("Filename"=w1466:path, "Row No"=w1476:i32, "Row Type Selector"=w1473:T3)
              n540 = call "Row_type_selector_string.vi"("Mode"=w1473) -> ("Output string"=w1472:string)
              n541 = call "Current_Filepath.vi"("Short_Name"="Res" ("Data Type"), "Filename in"=w1466, "Data Type"="Results") -> ("Filename Out"=w1467:path)  [unwired: 1 in, 1 out]
              n542 = Path To String(path=w1467) -> (string=w1484:string)
              n543 = Not A Number/Path/Refnum?(number/path/refnum=w1467) -> (NaN/Path/Refnum?=w1470:bool)
              n544 = Match Pattern(string=w1484, regular expression="-------" ("f")) -> (match substring=w1483:string)  [unwired: 4 out]
              n545 = Empty String/Path?(string/path=w1483) -> (empty?=w1471:bool)
              n546 = Format Into String(format string=" For Row  %d %s." ("Comment"), w1476, w1472) -> (resulting string=w1475:string)  [unwired: 2 in, 1 out]
              n547 = Compound Arithmetic op=AND(w1471, invert w1470) -> (w1469:bool)
              n548 = Select(t=w1467, s=w1469, f=path "") -> (s? t:f=w1482:path)
              n549 = call "Results_filename_checker.vi"("Warn if Already Exists"=FALSE, "Comment"=w1475, "Show Error handler"=w1487, "Results file"=w1482) -> ("Error String"=w1486:string, "cancelled"=w1478:bool, "Results file output"=w1463:path)  [unwired: 1 in, 1 out]
              n550 = Strip Path(path=w1463) -> (name=w1462:string)  [unwired: 1 out]
              n551 = Not(x=w1478) -> (.not. x?=w1474:bool)
              n552 = String To Path(string=w1462) -> (path=w1461:path)
              n553 = Bundle By Name(cluster=w1480, "Filename"=w1461) -> (w1479:T1)
            }
            frame "No Match", Default {
              n554 = Concatenate Strings(w1490, " Has not been programmed.\n" ("string")) -> (w1488:string)
            }
          }
        }
        n555 = local read "Edited Row"() -> (w1423:bool)
        n556 = And Array Elements(Boolean array=w1419) -> (logical AND=w1418:bool)
        n557 = Concatenate Strings(w1430) -> (w1428:string)
        n558 = Concatenate Strings(w1427, w1428) -> (w1422:string)
        n559 = Empty String/Path?(string/path=w1422) -> (empty?=w1425:bool)
        n560 = case shown="False" w1425 {
          tunnel: ["Open Front Panel" w1434] -> w1424
          tunnel: w1423 -> [_ w1435]
          frame False {
          }
          frame True {
            n561 = Select(t="Close Front Panel", s=w1435, f="End") -> (s? t:f=w1434:string)
          }
        }
      }
      frame "Open Front Panel" {
        w1497 = TRUE  # Front Panel Window:Open
        n562 = Current VI's Path() -> (path=w1498:path)
        n563 = call "Open_Close_Front_Panel.ph.vi"("openWindow (T)"=w1497, "VI path"=w1498) -> ()  [unwired: 1 in, 1 out]
        n564 = local write "Edited Row"(TRUE ("Editted Row")) -> ()
        n565 = local write "Execution Row"(w1494) -> ()
      }
      frame "What to do next?" {
        w1508 = ""
        w1507 = "[\r\n]"
        n566 = local read "Execution Row"() -> (w1506:T1)
        n567 = Wait Until Next ms Multiple(millisecond multiple=u32 100) -> ()  [unwired: 1 out]
        n568 = Unbundle By Name(w1506) -> ("Row Type Selector"=w1518:T3, "Specific Arguments"=w1515:string, "Extra Commands"=w1513:string)
        n569 = Not Equal?(x=Multi_run_mode."Blank Row" ("Mode"), y=w1518) -> (x != y?=w1516:bool)
        n570 = Compound Arithmetic op=OR("Edit in Excel", "OK") -> (w1502:bool)
        n571 = call "Replace_Character.vi"("Replace with"=w1508, "Input String"=w1515, "Search For"=w1507) -> ("Output string"=w1514:string)  [unwired: 1 out]
        n572 = call "Replace_Character.vi"("Replace with"=w1508, "Input String"=w1513, "Search For"=w1507) -> ("Output string"=w1512:string)  [unwired: 1 out]
        n573 = Compound Arithmetic op=AND(w1502, w1516) -> (w1510:bool)
        n574 = Bundle By Name(cluster=w1506, "Specific Arguments"=w1514, "Extra Commands"=w1512) -> (w1504:T1)
        n575 = case shown="False" "Edit in Excel" {
          tunnel: [w1526 "Close Front Panel"] -> w1509
          tunnel: w1510 -> [w1525 _]
          frame False {
            n576 = Select(t="Clean Up Row", s=w1525, f="What to do next?") -> (s? t:f=w1526:string)
          }
          frame True {
            n577 = Path To String(path="multirunFilepath") -> (string=w1529:string)
            n578 = Concatenate Strings("explorer " ("string"), w1529) -> (w1530:string)
            n579 = call <vilib>:"System Exec.vi"("command line"=w1530) -> ()  [unwired: 7 in, 4 out]
          }
        }
        n580 = Not Equal?(x=w1504, y=w1506) -> (x != y?=w1505:bool)
        n581 = case shown="True" w1505 {
          tunnel: w1504 -> [_ w1522]
          frame False {
          }
          frame True {
            n582 = local write "Execution Row"(w1522) -> ()
          }
        }
        n583 = Not(x="Edit in Excel") -> (.not. x?=w1503:bool)
        "Error Comments" <- w1511
      }
      frame "Clean Up Row" {
        n584 = call "Traverse_Control_Ch_Names.vi"("Mode"=T4."All Channel Names") -> ("Channel names"=w1540:string[])  [unwired: 1 in]
        n585 = call "Trav_Cluster_to_Row.vi"("Traverse line in"=w1535, "Row Number"=w1536, "Channel names"=w1540) -> ("Traverse line Out"=w1538:T1)  [unwired: 4 out]
      }
      frame "Close Front Panel" {
        w1544 = FALSE  # Front Panel Window:Open
        n586 = Current VI's Path() -> (path=w1545:path)
        n587 = call "Open_Close_Front_Panel.ph.vi"("openWindow (T)"=w1544, "VI path"=w1545) -> ()  [unwired: 1 in, 1 out]
      }
      frame "End" {
        n588 = local read "Edited Row"() -> (w1553:bool)
        n589 = case shown="True" w1553 {
          tunnel: w1552 -> [w1556 w1559]
          tunnel: [w1556 w1558] -> w1550
          tunnel: w1551 -> [_ w1557]
          frame False {
          }
          frame True {
            n590 = call "Traverse_Control_Ch_Names.vi"("Mode"=T4."All Channel Names") -> ("Channel names"=w1560:string[])  [unwired: 1 in]
            n591 = call "Trav_Cluster_to_Row.vi"("Traverse line in"=w1559, "Row Number"=w1557, "Channel names"=w1560) -> ("Traverse line Out"=w1558:T1)  [unwired: 4 out]
          }
        }
        n592 = local write "Error Comments"(w1554) -> ()
      }
    }
    "Traverse line Out" <- w8
  }
  "Execution Row Out" <- w2
  "Continue?" <- w1
